vi "AlliGator Conditional Menu Items.vi"(6 "Dataset Series?":bool, 7 "Help?":bool, 8 "Error In":errorcluster, 9 "Menu Item Path":string, 10 "Menu Item Tag":string, 11 "menu reference":refnum<k9>) -> (0 "Error Out":errorcluster, 1 "Quit?":bool, 2 "Message":string, 3 "AlliGator Actions":T1[](array[typedef]))   [LabVIEW 2021, in "AlliGator GUI.lvlib"]
doc: "Handles AlliGator menu items that are only responsive when AlliGator is idle."
uses:
  AlliGator GUI.lvlib
  Phasor/Phasor Calibration Type.ctl
  Action Engine/AlliGator Q Element.ctl
  Action Engine/AlliGator Q Event.ctl
  Image/Image Display Event.ctl
  Image/Image Control Refnum.ctl
  <vilib>/Utility/miscctls.llb/LVPoint32TypeDef.ctl
  Graphs/XY Graph/XY Graph Event.ctl
  Files/AlliGator FLI Dataset Type.ctl
  Files/AlliGator Load Dataset Options.ctl
  Files/AlliGator Select Folder Mode.ctl
  Files/AlliGator Folder Selection.ctl
  Files/AlliGator Export Dataset Options.ctl
  Globals, Variables, Constants/AlliGator Variables List.ctl
  Settings/AlliGator Settings List.ctl
  Fits/Decay Convolution/Decay Model.ctl
  Fits/Residual Type.ctl
  Fits/Non-linear Fitting Method v2.ctl
  Fits/Fit Calculation Method.ctl
  Fits/Non-linear Fitting Algorithm.ctl
  Files/Load-Save File Info.ctl
  AlliGator Windows List.ctl
  AlliGator Open Wndow Event Data.ctl
  GUI/Open VI Options.ctl
  Settings/AlliGator Settings Event.ctl
  Settings/AlliGator Settings Window Messages.ctl
  7dfe82a0-ef7a-4bbc-96a2-555d14fb2b04.vi
  Arrays/Signed Array Index.vi
  Variant/Variant to Data/Variant to Boolean.vi
  Action Engine/AlliGator Action Engine.lvlib
  Files/AlliGator Files.lvlib
  Globals, Variables, Constants/AlliGator Globals, Variables & Constants.lvlib
  Variant/Variant to Data/Variant to Data.lvlib
  Phasor/Phasor.lvlib
  Files/Files.lvlib
  Image/Image.lvlib
  Strings/Strings.lvlib
  Python Plugins API/AlliGator Python Plugins.lvlib
  Sound/Sound.lvlib
  Graphs/XY Graph/XY Graph Add-Ons.lvlib
  Settings/AlliGator Settings.lvlib
  Fits/Fits.lvlib
  GUI/GUI.lvlib
  Scripts/AlliGator Scripts.lvlib
  Fits/IRF(X)PSED/Fit Weights Type v2.ctl
  Fits/IRF(X)PSED/Decay Fit Options v4.ctl
panel:
  in  "Calibration Type":T3
  # "see the AlliGator License on the block diagram (Ctrl+E or Window:Show Block Diagram)"
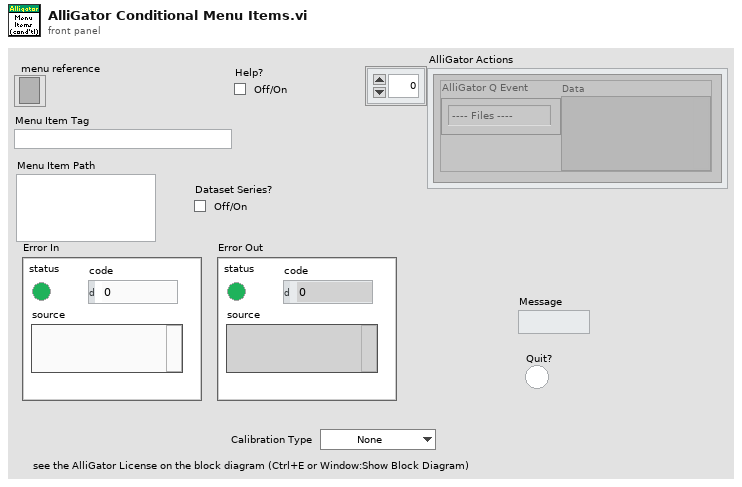
[diagram p1: front panel]
types:
  T1 = typedef "AlliGator Action Engine.lvlib/AlliGator Q Element.ctl" = cluster{"AlliGator Q Event":T2, "Data":variant}
  T2 = typedef "AlliGator Action Engine.lvlib/AlliGator Q Event.ctl" = enum16{"---- Files ----", "Files:Set Batch Export Files To Save", "Files:Set Dataset Loading & Pre-processing Options", "Files:Check #Frames in Dataset", "Files:Increment Frame Index", "Files:Open Mask Image", "Files:Open White Light Image", "Files:Open Single Dataset", "Files:New Folder of Folders Selected", "Files:Load File (all Types)_Scriptable", "Files:Move Flattened Series to Folders Series", "Files:Select Folder", "Files:Load FLI Dataset", "Files:Load Swiss SPAD 1 Dataset", "Files:Load Swiss SPAD 2 Dataset", "Files:Load .sdt FLI Dataset", "Files:Load .ptu FLI Dataset", "Files:Load .bin FLI Dataset", "Files:Load Single Gate Image Folder", "Files:Load I/m/phi Dataset (deprecated)", "Files:Load Single Image", "Files:Subtract Background File", "Files:Export FLI Dataset", "Files:Load HDF5 FLI Dataset", "Files:Set Destination File Path", "Files:Save Mask Image", "Files:Batch Conversion", "Files:New Folder Selected", "Files:Close FLI Dataset", "Files:Close FLI Dataset Series", "Files:Close White Light Image", "Files:Close Mask Image", "---- FLI Dataset ----", "FLI Dataset:Channel Arithmetic", "FLI Dataset:Export Average Lifetime Map as ASCII", "FLI Dataset:Export User-Defined Quantity Map as ASCII", "FLI Dataset:Python Function FLI Dataset Event", "FLI Dataset:ROI Analysis", "FLI Dataset:Tilted Logistic Square Gated IRF Characteristics Map", "FLI Dataset:Logistic Square Gated IRF Characteristics Map", "FLI Dataset:Square Gated IRF Characteristics Map", "FLI Dataset:Multi-ROI Single-Pixel Phasor Analysis", "FLI Dataset:Multi-ROI Single-Pixel NLSF Analysis", "FLI Dataset:All ROIs IRF Extraction", "FLI Dataset:All ROIs Decay Fit Non-Interactive (Fast + Individual IRF)", "FLI Dataset:All ROIs Phasor Analysis", "FLI Dataset:All ROIs Decay Fit", "FLI Dataset:Fluorescence Decay Statistics", "FLI Dataset:Update Decay Statistics Graph", "FLI Dataset:Get Decay from ROI", "FLI Dataset:All ROIs Average Lifetimes", "FLI Dataset:Save/Load Local IRFs", "FLI Dataset:Clear Local IRFs", "FLI Dataset:Phasor Calibration Maps (# Gates Series) Script", "FLI Dataset:Calibrated Phasor Map Series", "---- FLI Dataset Series ----", "FLI Dataset Series:Sum All Datasets in Series", "FLI Dataset Series:Add Dataset to Accumulated Dataset", "FLI Dataset Series:Display Accumulated Dataset", "FLI Dataset Series:Clear Dataset Series Sum", "FLI Dataset Series:Time-Series Analysis (NLSF)", "FLI Dataset Series:Time-Series Analysis (Phasor)", "---- Image ----", "Image:Update Image Profile Plots", "Image:Image Histogram Cursor Move", "Image:Image Histogram", "Image:Image Contrast", "Image:Set Image Histogram Cursor Move Flag", "Image:Clear Image Overlay", "Image:Use ROI as Search Area", "Image:Set ROI Diameter", "Image:Save Image Data as TIFF", "Image:Save Displayed Image with Overlay", "Image:Save Image Overlay Only", "Image:Save Image as Hot Pixel Mask", "Image:Change Source Image Color Palette", "Image:Copy Image to Clipboard", "Image:Source Image ROI Selection", "Image:Delete All ROIs", "Image:Delete All Unselected ROIs", "Image:Delete ROI", "Image:Merge All ROIs", "Image:Store ROI", "Image:Source Image ROI Storage", "Image:Export ROI Description to Notebook", "Image:Save ROI", "Image:Load ROI", "Image:Paste ROI Definition", "Image:Clear ROI", "Image:Identify ROIs in Mask Image", "Image:Create Complementary ROI", "Image:Create Contour ROI", "Image:Create ROI(s) from Pixels with Peak above Min_Scriptable", "Image:Create ROI(s) from Pixels with Intensity above Min_Scriptable", "Image:Compute ROI Statistics", "Image:Delete ROI(s) based on ROI Characteristics", "Image:Create ROI Grid", "Image:ROI to Individual Pixel ROIs", "Image:Python Function Source Image Event", "Image:Show Phasor Calibration Map ROI Centers", "Image:Convert ROI to Mask Image", "Image:Mouse Move", "Image:Mouse Up", "Image:Set Source Image Mouse Move Flag", "Image:Add Scale Bar Overlay", "Image:Delete Existing ROIs Option", "Image:Overlay ROI Median", "Image:Check Current ROI", "Image:Update True Pixel Value", "---- Decay ----", "Decay:Clear IRF/Reference Plot", "Decay:Add Decay to Graph", "Decay:Smoothen Plot", "Decay:Smoothen Plot Tail", "Decay:Average Selected Plots", "Decay:Extract IRF", "Decay:Optimal IRF Extraction", "Decay:Threshold IRF", "Decay:Fit to Model IRF", "Decay:Fit IRF to Square Gate", "Decay:Fit IRF to Logistic Square Gate", "Decay:Fit IRF to Tilted Logistic Square Gate", "Decay:Create Bounding Cursors Set", "Decay:Export Bounding Cursors Definition to Notebook", "Decay:Denoise Plot", "Decay:Compute Cumulative Function", "Decay:Use as Reference Decay", "Decay:Show Reference Decay/IRF", "Decay:Extrapolate Decay", "Decay:Create Head & Tail Bounding Cursors", "Decay:Store Cursor-defined Head & Tail Fractions", "Decay:Rebin Plot", "Decay:1-Normalize Decay", "Decay:[0-1]-Normalize Plot", "Decay:Straighten Decay", "Decay:Shift Decay", "Decay:Fold Decay", "Decay:Fit Decay", "Decay:Global Fit of Selected Decays", "Decay:Post Global Fit Script", "Decay:Add Global Fit Parameters to Graph", "Decay:Add Decay Parameter(s) to Plot (Graph)", "Decay:Export Decay to Phasor Graph", "Decay:Compute Average Lifetime", "Decay:Plot Convolution", "Decay:Graph Tip Strip Update", "---- Decay Statistics ----", "Decay Statistics:Tip Strip Update", "---- Intensity Time Trace ----", "Intensity Time Trace:Use File Timestamp", "Intensity Time Trace:Load Intensity Corrections File", "Intensity Time Trace:Clear Intensity Corrections File", "Intensity Time Trace:Tip Strip Update", "---- Phasor Plot ----", "Phasor Plot:Build Phasor Plot", "Phasor Plot:Change Phasor Plot Color Palette", "Phasor Plot:Adjust Phasor Plot Display Range", "Phasor Plot:Highlight Image ROI in Phasor Plot", "Phasor Plot:Save Phasor Plot Image with Overlay", "Phasor Plot:Export Complex Phasor Map", "Phasor Plot:Export Phasor Ratio Map", "Phasor Plot:Export Average Lifetime Map", "Phasor Plot:Compute Phase Lifetime Histogram", "Phasor Plot:Compute Phasor Ratio Histogram", "Phasor Plot:Compute Phase Lifetime vs Intensity Scatter Plot", "Phasor Plot:Weber 2-Component Decomposition", "Phasor Plot:Update Phasor Color Map Vertices", "Phasor Plot:Clear Phasor Overlay", "Phasor Plot:Use Segment Extremities as References", "Phasor Plot:Use UC/Segment Intersections as References", "Phasor Plot:Use UC/Principal Axis Intersections as References", "Phasor Plot:Use UC/Linear Fit Intersections as References", "Phasor Plot:Update Phasor Plot Reference", "Phasor Plot:Show Local Phasor Info in Phasor Plot", "Phasor Plot:Update Phasor Plot State", "Phasor Plot:Phasor Plot ROI Storage", "Phasor Plot:Phasor Plot ROI Selection", "Phasor Plot:Python Function Phasor Plot Event", "Phasor Plot:Overlay Phasor ROI, Ratio or Map in Source Image", "Phasor Plot:Compute Decay of Selected Phasors", "Phasor Plot:Phasor at Image Pixel", "Phasor Plot:Mouse Move", "Phasor Plot:Mouse Up", "Phasor Plot:Display Range Mouse Move", "Phasor Plot:Set Mouse Move Flag", "Phasor Plot:Update True Phasor Plot Value", "---- Phasor Graph ----", "Phasor Graph:Get Phasor Value", "Phasor Graph:Create New Phasor Plot Dialog", "Phasor Graph:Update Last Phasor Value", "Phasor Graph:Update Phasor (m, phi)", "Phasor Graph:Remove Single Phasor from Plot", "Phasor Graph:Add Single Phasor to Plot", "Phasor Graph:Remove Phasor Plot", "Phasor Graph:Remove Selected Phasor Plots", "Phasor Graph:Clear Phasor Data", "Phasor Graph:Clear Phasor Graph", "Phasor Graph:Cursor Move", "Phasor Graph:Draw Cursor Connecting Line", "Phasor Graph:Clear Cursor Connecting Line", "Phasor Graph:Find UC Intersection", "Phasor Graph:Use UC/Cursor-Defined Line Intersections", "Phasor Graph:Use Selected Plots Fitted Line/UC Intersections", "Phasor Graph:Use Selected Plots Principal Axis/UC Intersections", "Phasor Graph:Show Single Phasor", "Phasor Graph:Save Single Phasor Plot", "Phasor Graph:Save All Phasor Plots", "Phasor Graph:Load Phasor Plot(s)", "Phasor Graph:Phasor Multiplication", "Phasor Graph:Compute Average Phasor", "Phasor Graph:Compute Multiple Average Phasors (Selected Plots)", "Phasor Graph:Export Single Phasor Plot Phase Lifetimes", "Phasor Graph:Parameter 2 vs Parameter 1 Scatter Plot", "Phasor Graph:Use Cursor n Location", "Phasor Graph:Set Reference n to Current Phase Lifetime Value", "Phasor Graph:Set Reference n to Lifetime Value", "Phasor Graph:Set Cursor n Location", "Phasor Graph:Save Phasor Graph Image", "Phasor Graph:Update SEPL Plot", "Phasor Graph:Export Single Phasor Plot Data", "Phasor Graph:Export Selected Phasor Plots Data", "Phasor Graph:Python Function Phasor Graph Event", "Phasor Graph:Tip Strip Update", "---- Calibration ----", "Calibration:Set Calibration Type", "Calibration:Load/Save Phasor Calibration", "Calibration:Load/Save Phasor Calibration Series", "Calibration:Load/Save Phasor Calibration Map", "Calibration:Use as Calibration", "Calibration:Compute Optimal Calibration from Phasor References", "Calibration:Clear Phasor Calibration", "Calibration:Single Phasor Calibration Information", "Calibration:Use as Calibration Series", "Calibration:Use as Calibration Map", "Calibration:Clear Calibration Series", "Calibration:Phasor Calibration Series Information", "Calibration:Clear Calibration Map", "Calibration:Phasor Calibration Map Information", "Calibration:Apply Phasor Calibration", "Calibration:Update Single Plot Calibration", "Calibration:Update Multiple Plots Calibration", "Calibration:Clear Single Plot Calibration", "Calibration:Clear All Plots Calibrations", "Calibration:Clear Plot(s) Calibration(s)?", "---- Phasor Ratio ----", "Phasor Ratio:Clear Reference n", "Phasor Ratio:Toggle Selected Plot(s)  Lock to Reference 1", "Phasor Ratio:Use as Reference n", "Phasor Ratio:Send Reference n to Notebook", "Phasor Ratio:Toggle Selected Plot(s)  Lock to Reference 2", "Phasor Ratio:Compute Phasor Ratio at Mouse Location", "Phasor Ratio:Compute Phasor Plot's Average Phasor Ratio", "Phasor Ratio:Compute Time-Series Phasor Ratios", "Phasor Ratio:Fit Line to Phasor Ratio Plot", "Phasor Ratio:Save References", "Phasor Ratio:Load References", "Phasor Ratio:Update Phasor Reference 1", "Phasor Ratio:Update Phasor Reference 2", "Phasor Ratio:Move Cursor n to Reference n", "Phasor Ratio:Use as Phasor Reference 1 Lifetime", "Phasor Ratio:Use as Phasor Reference 2 Lifetime", "Phasor Ratio:Export Phasor Ratio Map as ASCII", "Phasor Ratio:Tip Strip Update", "---- Lifetime & Other Parameters Graph ----", "Lifetime:Compute Sliced Mean, SDV and CV Plots", "Lifetime:Plot Decay Shifts", "Lifetime:Plot Histogram", "---- Decay Fit Parameter Map ----", "Decay Fit Parameter Map:Export ROI NLSF Data as ASCII", "Decay Fit Parameter Map:Set Decay Fit Parameter Map Selection", "Decay Fit Parameter Map:Build Decay Fit Parameter Map", "Decay Fit Parameter Map:Change Decay Fit Parameter Map Color Palette", "Decay Fit Parameter Map:Export Decay Fit Parameter Map Data as ASCII", "Decay Fit Parameter Map:Export All Decay Fit Parameter Maps Data as ASCII", "Decay Fit Parameter Map:Selected Parameter Scatterplot", "Decay Fit Parameter Map:Parameter 2 vs Parameter 1 Scatterplot", "Decay Fit Parameter Map:Save Decay Fit Parameter Map Image", "Decay Fit Parameter Map:Save-Load IRFs & Fit Data", "Decay Fit Parameter Map:Update Local Decay Plots", "Decay Fit Parameter Map:Python Function Decay Fit Parameters Map Event", "Decay Fit Parameter Map:Overlay Decay Fit Parameter Map in Source Image", "Decay Fit Parameter Map:Selected Parameter vs Intensity Scatterplot", "Decay Fit Parameter Map:Mouse Up", "Decay Fit Parameter Map:Mouse Move", "Decay Fit Parameter Map:Display Range Mouse Move", "Decay Fit Parameter Map:Change Map Resolution", "Decay Fit Parameter Map:Variance Significance Maps", "Decay Fit Parameter Map:Fit Result Constraints Window", "---- Parameter Map ----", "Parameter Map:Export ROI Parameters Data as ASCII", "Parameter Map:Delete Parameter Map Set", "Parameter Map:Update Parameter List", "Parameter Map:Build Parameter Map", "Parameter Map:Change Parameter Map Color Palette", "Parameter Map:Export Parameter Map Data as ASCII", "Parameter Map:Export All Parameter Maps Data as ASCII", "Parameter Map:Selected Parameter Scatterplot", "Parameter Map:Parameter 2 vs Parameter 1 Scatterplot", "Parameter Map:Selected Parameter vs Intensity Scatterplot", "Parameter Map:Save Parameter Map Image", "Parameter Map:Save-Load IRFs & Parameter Maps (TODO)", "Parameter Map:Set Parameter Map Selection", "Parameter Map:Python Function Parameter Map Event", "Parameter Map:Overlay Parameter Map in Source Image", "Parameter Map:Update Local Decay Plots", "Parameter Map:Mouse Up", "Parameter Map:Mouse Move", "Parameter Map:Display Range Mouse Move", "---- Generic Graph ----", "Generic Graph:Generic XY Graph Event", "Generic Graph:Python Function XY Graph Event", "Generic Graph:New Plot", "Generic Graph:Save Plot", "Generic Graph:XY Plot Histogram", "Generic Graph:Set XY Graph Plot Name", "Generic Graph:Set Last Cursor Style", "Generic Graph:Tip Strip Update", "---- GUI ----", "GUI:Start Script", "GUI:Type of Displayed Image Changed", "GUI:Gate Image Slide Changed", "GUI:Show Busy Icon", "GUI:Show Busy Icon & Abort Button", "GUI:Hide Busy Icon", "GUI:Hide Busy Icon & Abort Button", "GUI:Abort", "GUI:End Script", "GUI:Start Timing", "GUI:End Timing", "GUI:Set State Indicator", "GUI:Send Parameters JSON Strings to Clipboard", "GUI:Set Gate Step", "GUI:Idle", "GUI:Initialization", "GUI:Quit", "GUI:Increment Dataset Index", "GUI:Set Dataset Index to -1", "GUI:Time Series Slider Moved", "GUI:Time Series Slider Changed", "GUI:Toggle Playback or Loop", "GUI:Playback Script", "GUI:Set Phasor Frequency", "GUI:Open Window", "GUI:Start Test Script", "GUI:End Test Script", "GUI:Set Verbose Mode", "GUI:Set Verbose Settings Mode", "DEBUG"}
  T3 = typedef "Phasor.lvlib/Phasor Calibration Type.ctl" = enum16{"None", "Single Phasor", "Phasor Series", "Phasor Map"}
  T4 = typedef "Image.lvlib/Image Display Event.ctl" = cluster{"Item Tag":string, "Image Control Refnum":T5, "Coords":T6, "Item Path":string}
  T5 = typedef "Image.lvlib/Image Control Refnum.ctl" = refnum<vi>
  T6 = typedef "LVPoint32TypeDef.ctl" = cluster{"Horizontal":i32, "Vertical":i32}
  T7 = typedef "XY Graph Add-Ons.lvlib/XY Graph Event.ctl" = cluster{"Item Tag":string, "XY Graph Refnum":refnum<vi>, "Coords":T6, "Item Path":string}
  T8 = typedef "AlliGator Files.lvlib/AlliGator Load Dataset Options.ctl" = cluster{"FLI Dataset Type":T9, "No Dialog?":bool, "File Path":path}
  T9 = typedef "AlliGator Files.lvlib/AlliGator FLI Dataset Type.ctl" = enum16{"HDF5 FLI Dataset", "Gate Image Folder", ".sdt FLI Dataset (Becker & Hickl)", ".ptu FLI Dataset (PicoQuant)", "SS1 FLI Dataset", "SS2 FLI Dataset", "I/m/phi Dataset", ".bin FLI Dataset (PicoQuant Binned)", ".bin FLI Dataset (Piccolo Binned)", ".mat FLI Dataset"}
  T10 = typedef "AlliGator Files.lvlib/AlliGator Folder Selection.ctl" = cluster{"Folder Selection Mode":T11, "Folder Path":path}
  T11 = typedef "AlliGator Files.lvlib/AlliGator Select Folder Mode.ctl" = enum16{"Select Gate Folder", "Select Folder of Gate Folders", "Select Folder of SwissSPAD 2 Datasets", "Select Folder of .sdt FLI Datasets (Becker & Hickl)", "Select Folder of .ptu FLI Datasets (PicoQuant)", "Select Folder of .bin FLI Datasets (PicoQuant Binned)", "Select Folder of .bin FLI Datasets (Piccolo Binned)", "Select Folder of HDF5 FLI Datasets"}
  T12 = typedef "AlliGator Files.lvlib/AlliGator Export Dataset Options.ctl" = cluster{"Destination File Type":string, "Dialog?":bool}
  T13 = typedef "AlliGator Globals, Variables & Constants.lvlib/AlliGator Variables List.ctl" = enum16{"---- GUI ----", "GUI:Initialization Status", "GUI:State Indicators Refnum", "GUI:Original AlliGator Menu Items", "GUI:Current Action Loop State", "GUI:Script in progress", "GUI:Playback", "GUI:Loop Playback", "GUI:Search ROI Used", "GUI:Search ROI", "Decay Graph Max Legend Size", "Intensity Graph Max Legend Size", "Decay Statistics Graph Max Legend Size", "Phasor Graph Max Legend Size", "Phasor Ratio Graph Max Legend Size", "Lifetime Graph Max Legend Size", "---- Files ----", "Files:Export Dataset Frames as Individual Files", "Files:Show Batch Export Help Balloons", "Files:Frames in Dataset", "Files:ptu File Frame Start Indices", "Files:Current Frame in Dataset", "Files:Current Frame Timestamp", "Files:Dataset Loaded", "Files:Dataset Metadata", "Files:Dataset Channel", "Files:Dataset Data Description", "Files:Background Dataset Metadata", "Files:Background Dataset Channel", "Files:Background Dataset Data Description", "Files:Background File Subtraction", "Files:Background File Path", "Files:Background File Pile-up Correction", "Files:Background File Pixel Well Capacity", "Files:Background File Scaling Factor", "Files:Current Dataset Load Settings", "Files:Dataset Path", "Files:ICCD-specific Information", "Files:Macrotime Gate Separation", "------ Python Plugins ------", "Python Plugins:Information", "Python Plugins:Python Session", "Python Plugins:Valid Python Session?", "---- Source Image ----", "Source Image:ROIs", "Source Image:Current ROI", "Source Image:ROI Event Refnum", "X_Source Image:Display Range", "X_Source Image:Palette Information", "X_Source Image:Type of Displayed Image", "X_Time Gate Slider", "Source Image:Palette List", "Source Image:Scale", "Source Image:ROI Overlay Color", "Source Image:Overlay to Erase", "Source Image:Is Displayed Image Accumulated", "Source Image:White Light Image Modified", "Source Image:Mask Image Modified", "---- Image Profile Window ----", "Image Profile:Window Event Refnum", "Image Profile:IntensityType", "Image Profile:Intensity Average Type", "Image Profile:Intensity-weighted SDV", "Image Profile:Box Profile Type", "Image Profile:Window Open", "Image Profile:Plotted Fit Parameter", "------ Phasor Graph -------", "Phasor Graph:Show Line", "---- Phasor Plot ---", "Phasor Plot:Parameters Changed", "Phasor Plot:FLI Dataset Modified since last Calculation", "Phasor Harmonics Data", "Selected Phasor Harmonics", "Phasor Harmonic Manager Event Refnum", "Phasor Plot:ROIs", "Phasor Plot:Current ROI", "Phasor Plot:ROI Event Refnum", "Phasor Plot:Image Reference Points", "Phasor Plot:Computed", "Phasor Plot:Palette Information", "Phasor Plot:Palette List", "Phasor Plot:Phasor Ratio Palette Information", "Phasor Plot:Phasor Ratio Palette List", "Phasor Plot:Image Scale", "Phasor Plot:Image Overlay to Erase", "Phasor Plot:Image Elements to Update", "Phasor Plot:Current Calculation Parameters", "Phasor Plot:Current Calibration Options", "Phasor Plot:Reset Cumulated Phasor Plot", "Phasor Plot:Reference 1", "Phasor Plot:Lifetime Reference 1", "Phasor Plot:Reference 1 Frequency", "Phasor Plot:Reference 2", "Phasor Plot:Lifetime Reference 2", "Phasor Plot:Reference 2 Frequency", "---- Decay Analysis ----", "Number of Selected Decays to Fit", "LS Fit Results", "LAR Fit Results", "BS Fit Results", "Last Decay Max - Min", "Best Fit Parameters", "Best Fit Parameter Names", "Actual Size X", "Actual Size Y", "Binning X", "Binning Y", "Actual # Gates", "Dataset Number", "Gates to...", "Gates Skipped", "Gates to keep", "Gate Step", "Gate Separation", "Reversed Gates", "Pile-up Correction", "Pixel Well Capacity", "Background Subtracted", "Background Subtraction Method", "Background Definition Range", "Background File (deprecated)", "Number of Dataset Accumulated", "Array of Accumulated Dataset Paths", "Do Averaged Datasets", "Destination File Path", "Process Plot Target", "Use 1/D as Phasor Frequency", "---- Decay Fit Parameter Map -----", "Decay Fit Parameter Map:Palette Information", "Decay Fit Parameter Map:Palette List", "Decay Fit Parameter Map:X Resolution", "Decay Fit Parameter Map:Y Resolution", "Decay Fit Parameter Map:Use Decay Fit Result Constraints", "Decay Fit Parameter Map:Decay Fit Result Constraints", "Decay Fit Parameter Map:Decay Fit Result Constraints Applied", "---- Parameter Map ----", "Parameter Map:Palette Information", "Parameter Map:Palette List", "------- Local Decay Window ---------", "Local Decay Graph Window:Event Refnum", "Local Decay Graph Window:Use normalized IRF for convolution", "----- Miscellaneous ----", "Misc:Skippable Dialog Windows Status"}
  T14 = typedef "Fits.lvlib/Decay Fit Options v4.ctl" = cluster{"Show Fit Residuals":bool, "Fit Model":T15, "Residual Type":T16, "Max Decay Percentile":dbl, "Min Decay Percentile":dbl, "Show Full Decay":bool, "Weights":T17, "Fitting Method":T18, "Compute Parameter Uncertainties":bool, "Periodic Boundaries":bool, "Model Calculation":T19, "Period":dbl[unit], "Termination Criteria":cluster{"Max Iterations":i32, "Max Function Calls":i32, "Max Time":dbl[unit], "Function Tolerance":dbl, "Parameter Tolerance":dbl, "Gradient Tolerance":dbl, "Min Lambda":dbl, "Max Lambda":dbl, "Initial Tick Count":u32}, "Offset Resolution":dbl[unit], "Use Local IRF":bool, "Fitting Algorithm":T20, "Show Confidence Interval ":bool, "Confidence Level":dbl}
  T15 = typedef "Fits.lvlib/Decay Model.ctl" = enum16{"1-Exponential", "2-Exponentials"}
  T16 = typedef "Fits.lvlib/Residual Type.ctl" = enum16{"Standard", "Normalized", "Reduced"}
  T17 = typedef "Fits.lvlib/Fit Weights Type v2.ctl" = enum16{"Unweighted", "1/Variance (Neyman)", "1/Variance (Pearson)", "Best of All"}
  T18 = typedef "Fits.lvlib/Non-linear Fitting Method v2.ctl" = enum16{"Least Square", "Least Absolute Residual", "Bisquare", "MLE", "-", "Best of All"}
  T19 = typedef "Fits.lvlib/Fit Calculation Method.ctl" = enum16{"Simulation", "Convolution", "Integration"}
  T20 = typedef "Fits.lvlib/Non-linear Fitting Algorithm.ctl" = enum16{"Levenberg-Marquardt", "Trust-Region Dogleg"}
  T21 = typedef "AlliGator Settings.lvlib/AlliGator Settings List.ctl" = enum16{"GUI:Visible Settings Tab", "GUI:Last Run Version", "Source Image:Use Image Histogram for Contrast", "Source Image:Low Count Pixels Rejection Options", "Source Image:High Count Pixels Rejection Options", "Source Image:Use Image Brightness", "Source Image:Blend Overlay with Image Background", "Source Image:Use Fixed ROI Diameter", "Source Image:ROI Diameter", "Source Image:ROI Center Color", "Source Image:Peak Threshold", "Source Image:Intensity Threshold", "Source Image:Image Binning Options", "Source Image:Image Smoothing Options", "Source Image:Image Histogram Active", "Source Image:Invert Binary Mask", "Source Image:Hot Pixel Removal", "Source Image:Overlay Analyzed ROI Center", "Source Image:Auto-Adjust Contrast", "Source Image:Histogram Lower Percentile", "Source Image:Histogram Upper Percentile", "Source Image:Save Source Image", "Source Image:Scale Bar Options", "Source Image:Image Resolution (Pixel Size)", "Source Image:Flatfield Correction", "Source Image:Show Dead Left Columns Correction", "Source Image:Dead Left Columns Correction", "Source Image:Image Pre-Processing Operations Order", "Source Image:Overlay ROI Median", "Source Image:Median Overlay Color", "Data Information:Gate Width", "Data Information:Nanotime Gate Separation", "Data Information:Macrotime Gate Separation", "Data Information:Gate Step", "Data Information:# Gates", "Data Information:Gate Image Exposure", "Data Information:Gate Image Integration", "Data Information:Gates to Skip", "Data Information:Gates to Keep", "Data Information:Define Gates to", "Data Information:Channel Name", "Data Information:Available Channel Names", "Data Information:Channel Arithmetic", "Data Information:Background File Subtraction", "Data Information:Background File", "Data Information:Background Scaling Factor", "Data Information:Background Pile-up Correction", "Data Information:Background Pixel Well Capacity", "Data Information:Laser Period", "Data Information:SYNC Period", "Data Information:Pile-up Correction", "Data Information:Pixel Well Capacity", "Data Information:Dataset Scaling Factor", "Fluorescence Decay_Decay Pre-Processing:Reverse Gates", "Fluorescence Decay_Decay Pre-Processing:Verbose Decay Pre-Processing", "Fluorescence Decay_Decay Pre-Processing:Use Decay Pre-Processing", "Fluorescence Decay_Decay Pre-Processing:Background Subtraction", "Fluorescence Decay_Decay Pre-Processing:Background Definition Range", "Fluorescence Decay_Decay Pre-Processing:Baseline Subtraction Method", "Fluorescence Decay_Decay Pre-Processing:Decay Pre-Processing Operations Order", "Fluorescence Decay_Decay Pre-Processing:Smoothing Parameter", "Fluorescence Decay_Decay Pre-Processing:Shift Decay", "Fluorescence Decay_Decay Pre-Processing:Decay Shift Parameters", "Fluorescence Decay_Decay Pre-Processing:Fold Decay", "Fluorescence Decay_Decay Pre-Processing:# Folds", "Fluorescence Decay_Decay Pre-Processing:1-Normalize Decay", "Fluorescence Decay_Decay Pre-Processing:[0-1]-Normalize Decay", "Fluorescence Decay_Decay Pre-Processing:Smoothen Decay", "Fluorescence Decay_Decay Pre-Processing:Extrapolate Decay", "Fluorescence Decay_Decay Pre-Processing:Use Periodicity", "Fluorescence Decay_Decay Pre-Processing:Use Cursors", "Fluorescence Decay_Decay Pre-Processing:Tail Fraction", "Fluorescence Decay_Decay Pre-Processing:Head Fraction", "Fluorescence Decay_Decay Pre-Processing:Additional Points", "Fluorescence Decay_Decay Pre-Processing:Straighten Decay", "Fluorescence Decay_Decay Pre-Processing:Constant Background", "Fluorescence Decay_Decay Pre-Processing:Pixel-Normalize Decay", "Fluorescence Decay_Advanced Analysis:Extract IRF instead of Decay", "Fluorescence Decay_Advanced Analysis:IRF Extraction Options", "Fluorescence Decay_Advanced Analysis:IRF Optimization Options", "Fluorescence Decay_Advanced Analysis:Square Pulse Options", "Fluorescence Decay_Advanced Analysis:IRF Order", "Fluorescence Decay_Advanced Analysis:IRF Time Constants", "Fluorescence Decay_Advanced Analysis:Wavelet Analysis Options", "Fluorescence Decay_Advanced Analysis:Average Lifetime Options", "Fluorescence Decay_Fit Options:Fit Options", "Fluorescence Decay_Fit Options:Use Legacy Fitting Approach", "Fluorescence Decay_Fit Options:Use Data Information Laser Period", "Fluorescence Decay_Fit Parameters:Displayed Fit Parameters", "Fluorescence Decay_Fit Parameters:Fit Parameter Constraints", "Fluorescence Decay_Fit Parameters:Export Tabulated Results", "Fluorescence Decay_Fit Parameters:MLE Baseline Offset Type", "Fluorescence Decay_Fit Parameters:MLE Baseline Offset", "Fluorescence Decay_Fit Parameters:Guess Parameter Names", "Fluorescence Decay_Fit Parameters:Guess Parameter Values", "Fluorescence Decay_Fit Parameters:Guess Parameters Options", "Fluorescence Decay_Fit Parameters:Optimal Offset Selection Criterion", "Fluorescence Decay_Styles:Show Last Decay Only", "Fluorescence Decay_Styles:Decay Graph Color Array", "Fluorescence Decay:Decay Graph Active", "Fluorescence Decay Statistics:Min Peak Value", "Fluorescence Decay Statistics:Reject Low Decay Peak Pixels", "Fluorescence Decay Statistics:Reject High Decay Peak Pixels", "Fluorescence Decay Statistics:Max Peak Value", "Time Traces:Use File Timestamp", "Time Traces:Time Step", "Time Traces:Use Intensity Correction File", "Time Traces:Intensity Correction File", "Phasor Plot:Phasor Plot Smoothing Options", "Phasor Plot:Phasor Plot Size", "Phasor Plot:Phasor Plot Graphics Options", "Phasor Plot:Cumulative Phasor Plot", "Phasor Plot:Use Phasor Brightness", "Phasor Plot:Blend Overlay with Phasor Background", "Phasor Plot:Save Phasor Plot", "Phasor Plot:Show References", "Phasor Plot:Phasor Ratio Decay Range", "Phasor Plot:Exponential Fading", "Phasor Plot:Phasor Ratio Reference Colors", "Phasor Plot:Reference Radius", "Phasor Plot:Show Color Map Vertices", "Phasor Plot:Phasor Plot Active", "Phasor Plot:Phasor Ratio Color Map Type", "Phasor Plot:Phasor Ratio Color Map", "Phasor Plot:Phasor Ratio Display Range", "Phasor Plot:Selected Image ROI(s)", "Phasor Plot:All Image ROIs", "Phasor Plot:Selected Phasor Plot ROI(s)", "Phasor Plot:All Phasor Plot ROIs", "Phasor Plot:Phasor Ratio Color-Coded Quantity", "Phasor Plot:Store Phasor Harmonics", "Phasor Plot:Draw Reference Segment", "Phasor Plot:User-Defined Quantity", "Phasor Plot:Color Scale High Color", "Phasor Plot:Color Scale Low Color", "Phasor Plot:Intensity-weighted Phasor Plot", "Phasor Graph:Phasor Frequency", "Phasor Graph:Phasor Ratio Type", "Phasor Graph:Pixel-level Phasor Computation", "Phasor Graph:Save Phasor Graph", "Phasor Graph:Phasor Graph Active", "Phasor Graph:Phasor SDV Options", "Phasor Graph:Intensity-weighted Phasor Graph", "Phasor Graph:Define Shortest Lifetime as", "Phasor Calibration:Use Backup Calibration if needed", "Phasor Calibration:Backup Calibration Type", "Phasor Calibration:Calibration Type", "Phasor Calibration:Calibration Lifetime", "Phasor Calibration:Calibration Map Algorithm", "Single-Exponential Phasor Locus (SEPL):Gate Parameters", "Single-Exponential Phasor Locus (SEPL):User-defined Gate", "Single-Exponential Phasor Locus (SEPL):User-defined IRF", "Single-Exponential Phasor Locus (SEPL):Phasor Parameters", "Single-Exponential Phasor Locus (SEPL):Decay & IRF Parameters", "Single-Exponential Phasor Locus (SEPL):Display Parameters", "Lifetime Analysis:Decay Analysis Parameters", "Lifetime Analysis:Lifetime Map Active", "Plugins:Python Settings", "Miscellaneous:Verbose Mode", "Miscellaneous:Beep after Script", "Miscellaneous:Saved Image File Format", "Miscellaneous:Exported Gate Image Settings", "Miscellaneous:Include Loading in Timing", "Miscellaneous:Verbose Settings Mode", "Miscellaneous:Histogram Options", "Miscellaneous:Beep on Error", "Miscellaneous:# Logical Processors Used", "Miscellaneous:ROI Description Max Characters", "Miscellaneous:Verbose Error Mode", "Miscellaneous:Transparent Mask Color"}
  T22 = typedef "Files.lvlib/Load-Save File Info.ctl" = cluster{"Load/Save":bool, "File Path":path}
  T23 = typedef "AlliGator GUI.lvlib/AlliGator Open Wndow Event Data.ctl" = cluster{"AlliGator Windows":T24, "Open Window Options":T25}
  T24 = typedef "AlliGator GUI.lvlib/AlliGator Windows List.ctl" = enum16{"AlliGator Window", "Settings Window", "Notebook Window", "Dataset Information Window", "Source Image ROI Manager Window", "Phasor Plot ROI Manager Window", "Phasor Harmonic Manager Window", "Histogram Window", "Image Profile Window", "Local Decay Window", "About Window", "Batch Conversion Window", "Shot Noise Influence on Average Lifetime", "Fit Method Benchmark", "Camera Noise Influence on Lifetime", "AlliGator Alias Definition", "Fit Result Constraints Window"}
  T25 = typedef "GUI.lvlib/Open VI Options.ctl" = cluster{"Bring To Front (T)":bool, "Start Hidden? (F)":bool, "Activate? (T)":bool}
  T26 = typedef "AlliGator GUI.lvlib/AlliGator Ctrl Refnums.ctl" = cluster{"Other AlliGator Ctrl Refnums":T27, "Phasor Plot Ctrl Refnums":T28, "Phasor Graph Ctrl Refnums":T29, "Dataset Control Refnums":T30, "Registered Events Ctrl Refnums":T31, "Image Histogram Ctrl Refnums":T32, "Decay Fit Map Ctrl Refnums":T33, "Parameter Map Ctrl Refnums":T34}
  T27 = typedef "AlliGator GUI.lvlib/AlliGator Other Ctrl Refnums.ctl" = cluster{"State Indicators":refnum<vi>, " Progress Bar":refnum<vi>, "Decay Graph Active":refnum<vi>, "Decay Statistics Bin":refnum<vi>, "Time Step":refnum<vi>, "Use File Timestamp":refnum<vi>, "Tab Control":refnum<vi>, "CPU":refnum<vi>, "Abort Fit":refnum<vi>, "Dataset File/Folder Path":refnum<vi>, "Abort ROI Creation":refnum<vi>, "Event LED":refnum<vi>, "Dataset File/Folder Path 2":refnum<vi>, "Dataset File/Folder Path 3":refnum<vi>, "Dataset File/Folder Path 4":refnum<vi>, "Dataset File/Folder Path 5":refnum<vi>, "Dataset File/Folder Path 6":refnum<vi>, "Dataset File/Folder Path 7":refnum<vi>, "Dataset File/Folder Path 8":refnum<vi>, "Dataset File/Folder Path 9":refnum<vi>, "Dataset File/Folder Path 10":refnum<vi>, "Dataset File/Folder Path 11":refnum<vi>}
  T28 = typedef "AlliGator GUI.lvlib/AlliGator Phasor Plot Ctrl Refnums.ctl" = cluster{"Phasor Ratio":refnum<vi>, "Modulus Lifetime":refnum<vi>, "Phasor at cursor (m, phi)":refnum<vi>, "Phase Lifetime":refnum<vi>, "Phasor at cursor (g, s)":refnum<vi>, "Phasor Plor Average Lifetime":refnum<vi>, "Phasor Plot Active":refnum<vi>, "Save Phasor Plot":refnum<vi>, "Image Overlay Color":refnum<vi>, "Phasor Plot Color Scale":refnum<vi>, "Reference 1 Button":refnum<vi>, "Reference 2 Button":refnum<vi>, "True Phasor Plot Value":refnum<vi>}
  T29 = typedef "AlliGator GUI.lvlib/AlliGator Phasor Graph Ctrl Refnums.ctl" = cluster{"Phasor Ratio":refnum<vi>, "Modulus Lifetime":refnum<vi>, "Phasor at cursor (m, phi)":refnum<vi>, "Phase Lifetime":refnum<vi>, "Phasor at cursor (g, s)":refnum<vi>, "Phasor Graph Average Lifetime":refnum<vi>, "Phasor Graph Active":refnum<vi>, "Save Phasor Graph":refnum<vi>, "Phasor Frame Slide":refnum<vi>, "Single Step Phasor":refnum<vi>, "Calibration Type":refnum<vi>, "Show Line":refnum<vi>, "Phase Lifetime 1":refnum<vi>, "Phase Lifetime 2":refnum<vi>, "Phasor Graph Frequency":refnum<vi>, "Phasor Reference 1 Control":refnum<vi>, "Phasor Reference 2 Control":refnum<vi>, "Calibration Lifetime":refnum<vi>, "Phase Lifetime SDV":refnum<vi>, "Average Lifetime SDV":refnum<vi>, "Phasor Ratio SDV":refnum<vi>, "Modulus Lifetime SDV":refnum<vi>}
  T30 = typedef "AlliGator GUI.lvlib/AlliGator Dataset Ctrl Refnums.ctl" = cluster{"Current Data":refnum<vi>, "Gate Image Slide":refnum<vi>, "Time Point Slide":refnum<vi>, "Current Time Stamp":refnum<vi>, "Save Image":refnum<vi>, "Displayed Image":refnum<vi>, "Overlay Mode":refnum<vi>, "Phasor Overlay Color":refnum<vi>, "Image Color Scale":refnum<vi>, "Use ROI as Search Area":refnum<vi>, "Source Image ROI Color":refnum<vi>, "True Pixel Value":refnum<vi>}
  T31 = typedef "AlliGator GUI.lvlib/AlliGator Registered Events Ctrl Refnums.ctl" = cluster{"Time Point Slider":refnum<vi>, "Phasor Plot Display Range":refnum<vi>, "Decay Graph":refnum<vi>, "Decay Statistics Graph":refnum<vi>, "Intensity Time Trace":refnum<vi>, "Phasor Graph":refnum<vi>, "Phasor Ratio Graph":refnum<vi>, "Lifetime Graph":refnum<vi>, "Phasor Plot Display":refnum<vi>, "Source Image Display":refnum<vi>, "Decay Fit Parameter Map Display Range":refnum<vi>, "Decay Fit Parameter Map Display":refnum<vi>, "Parameter Map Display Range":refnum<vi>, "Parameter Map Display":refnum<vi>, "Phasor Plot Display Range":refnum<vi>}
  T32 = typedef "AlliGator GUI.lvlib/AlliGator Image Histogram Control Refnums.ctl" = cluster{"Image Histogram":refnum<vi>, "Image Histogram Options":refnum<vi>, "Image Histogram Active":refnum<vi>, "Image Histogram Upper Percentile":refnum<vi>, "Image Histogram Lower Percentile":refnum<vi>, "Auto-Adjust Contrast":refnum<vi>}
  T33 = typedef "AlliGator Decay Fit Parameter Map.lvlib/AlliGator Decay Fit Map Control Refnums.ctl" = cluster{"Decay Fit Parameter Map Color Scale":refnum<vi>, "Decay Fit Parameter":refnum<vi>, "Max Parameter":refnum<vi>, "Min Parameter":refnum<vi>, "Decay Fit Parameter Map Display":refnum<vi>, "Decay Fit Parameter Map Display Range":refnum<vi>, "Decay Parameter Map X":refnum<vi>, "Decay Parameter Map Y":refnum<vi>, "Decay Parameter Map Value":refnum<vi>}
  T34 = typedef "AlliGator Parameter Map.lvlib/AlliGator Parameter Map Control Refnums.ctl" = cluster{"Parameter Map Color Scale":refnum<vi>, "Map Parameter":refnum<vi>, "Max Parameter":refnum<vi>, "Min Parameter":refnum<vi>, "Parameter Map Display":refnum<vi>, "Parameter Map Display Range":refnum<vi>, "Parameter Map Set":refnum<vi>, "Parameter Map X":refnum<vi>, "Parameter Map Y":refnum<vi>, "Parameter Map Value":refnum<vi>}
  T35 = typedef "AlliGator Scripts.lvlib/AlliGator Series Analysis Type.ctl" = enum16{"Current ROI (Fixed)", "All ROIs (Fixed)", "Sequential ROIs"}
  T36 = typedef "AlliGator Settings.lvlib/AlliGator Settings Event.ctl" = cluster{"AlliGator Settings Message":T37, "Sender":string, "Control Label":string, "Data":variant}
  T37 = typedef "AlliGator Settings.lvlib/AlliGator Settings Window Messages.ctl" = enum16{"Idle", "Subscribe", "Unsubscribe", "Refresh Parameter", "Refresh All Parameters", "Quit"}
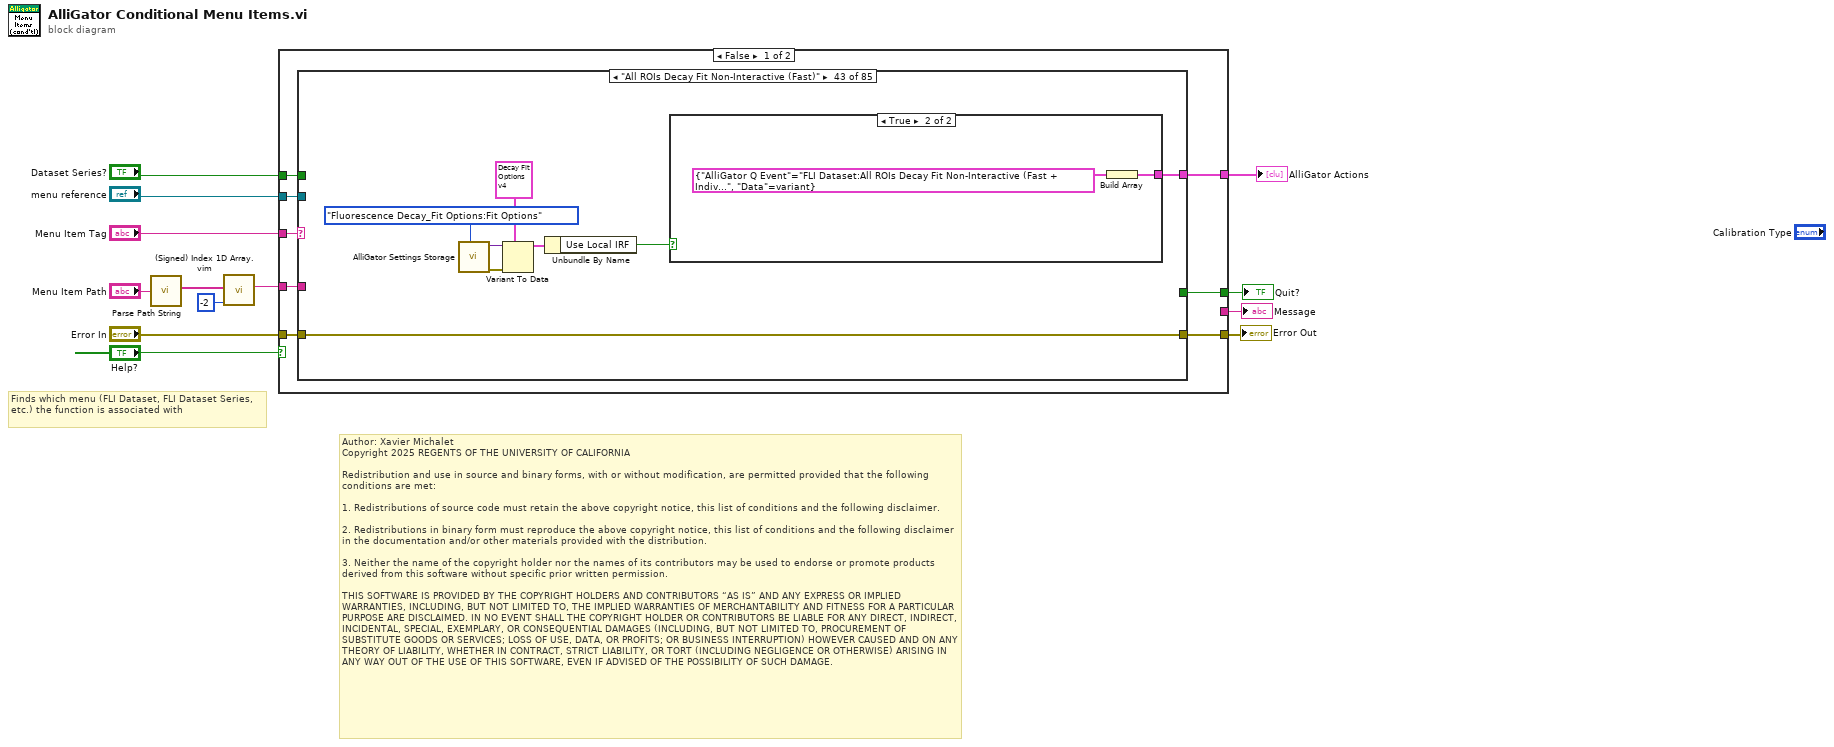
[diagram p0: block diagram]
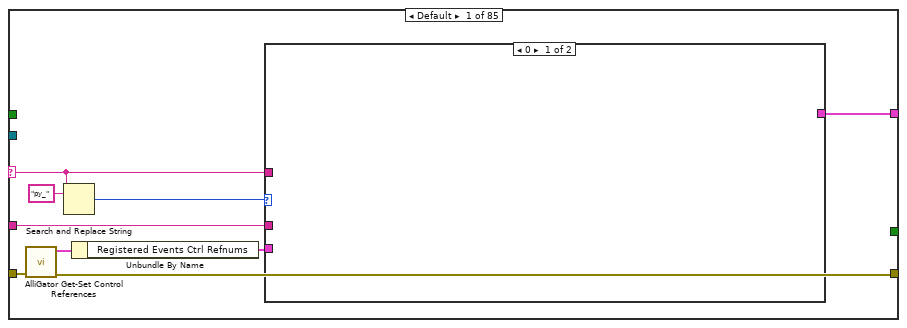
[diagram p2: hidden frame]
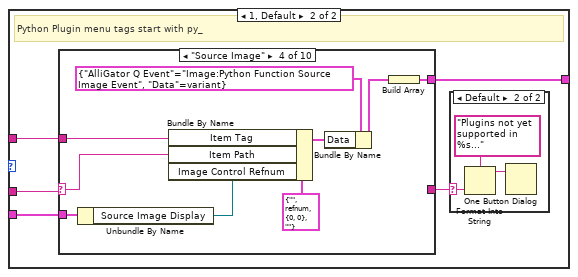
[diagram p3: hidden frame]
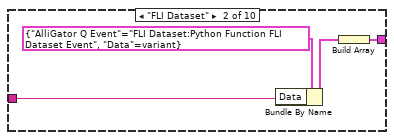
[diagram p6: hidden frame]
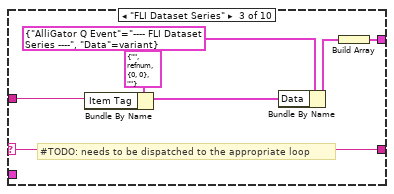
[diagram p7: hidden frame]
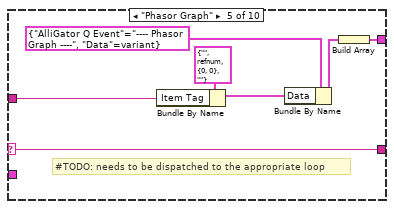
[diagram p8: hidden frame]
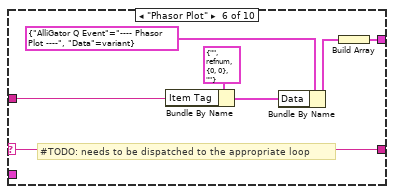
[diagram p9: hidden frame]
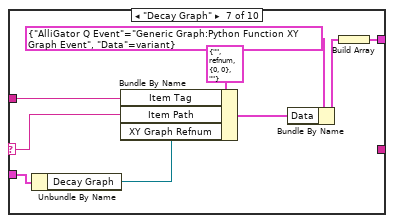
[diagram p10: hidden frame]
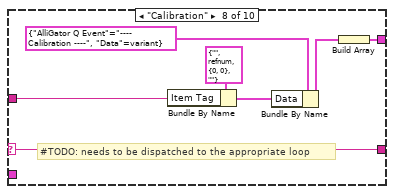
[diagram p11: hidden frame]
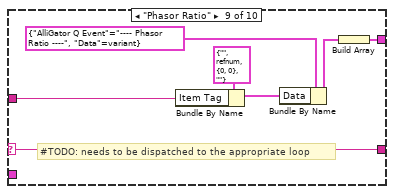
[diagram p12: hidden frame]
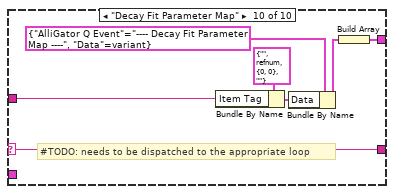
[diagram p13: hidden frame]
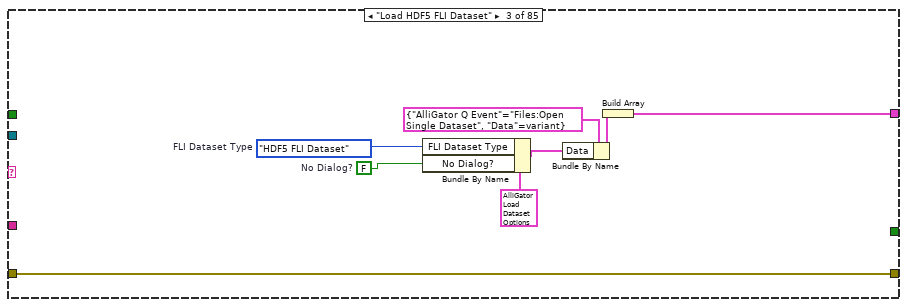
[diagram p15: hidden frame]
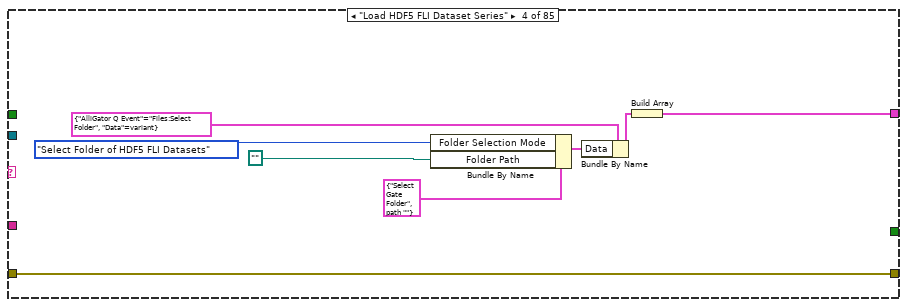
[diagram p16: hidden frame]
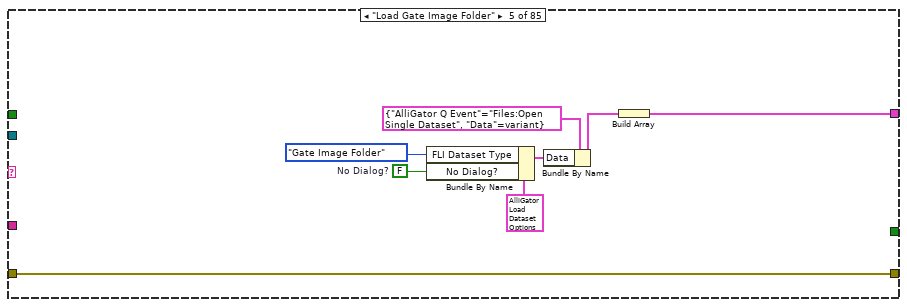
[diagram p17: hidden frame]
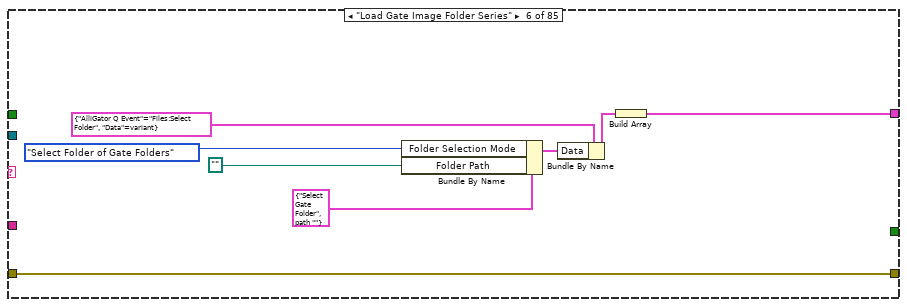
[diagram p18: hidden frame]
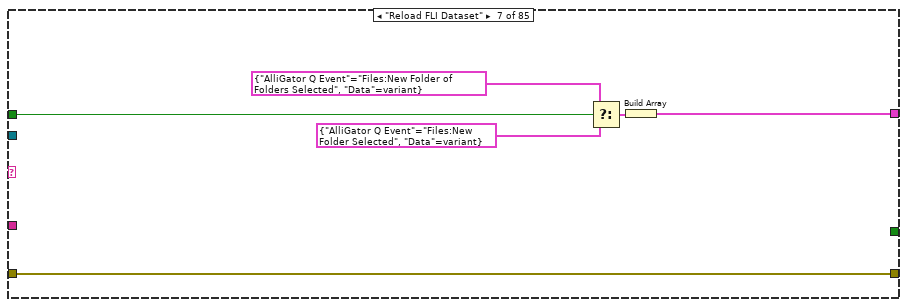
[diagram p19: hidden frame]
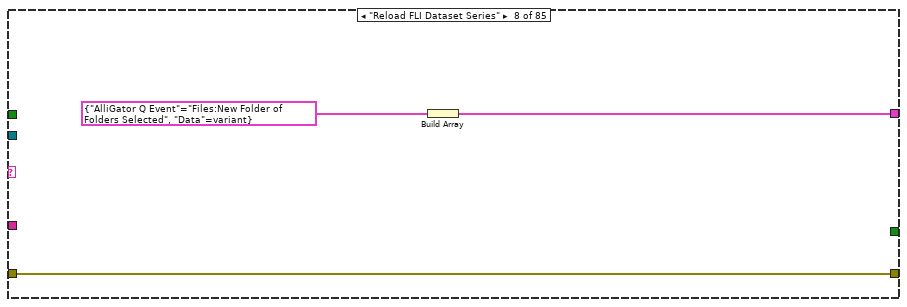
[diagram p20: hidden frame]
diagram:
  # "Author: Xavier Michalet\nCopyright 2025 REGENTS OF THE UNIVERSITY OF CALIFORNIA\n\nRedistribution and use in source and binary forms, with or without modification, are permitted provided that the following conditions are met:\n\n1. Redistributions of source code must retain the above copyright notice, this list of conditions and the following disclaimer.\n\n2. Redistributions in binary form must reproduce the above copyright notice, this list of conditions and the following disclaimer in the documentation and/or other materials provided with the distribution.\n\n3. Neither the name of the copyright holder nor the names of its contributors may be used to endorse or promote products derived from this software without specific prior written permission.\n\nTHIS SOFTWARE IS PROVIDED BY THE COPYRIGHT HOLDERS AND CONTRIBUTORS “AS IS” AND ANY EXPRESS OR IMPLIED WARRANTIES, INCLUDING, BUT NOT LIMITED TO, THE IMPLIED WARRANTIES OF MERCHANTABILITY AND FITNESS FOR A PARTICULAR PURPOSE ARE DISCLAIMED. IN NO EVENT SHALL THE COPYRIGHT HOLDER OR CONTRIBUTORS BE LIABLE FOR ANY DIRECT, INDIRECT, INCIDENTAL, SPECIAL, EXEMPLARY, OR CONSEQUENTIAL DAMAGES (INCLUDING, BUT NOT LIMITED TO, PROCUREMENT OF SUBSTITUTE GOODS OR SERVICES; LOSS OF USE, DATA, OR PROFITS; OR BUSINESS INTERRUPTION) HOWEVER CAUSED AND ON ANY THEORY OF LIABILITY, WHETHER IN CONTRACT, STRICT LIABILITY, OR TORT (INCLUDING NEGLIGENCE OR OTHERWISE) ARISING IN ANY WAY OUT OF THE USE OF THIS SOFTWARE, EVEN IF ADVISED OF THE POSSIBILITY OF SUCH DAMAGE."
  # "Finds which menu (FLI Dataset, FLI Dataset Series, etc.) the function is associated with"
  n1 = call "Parse Path String.vi"("Path in"="Menu Item Path") -> ("Folder Hierarchy"=w6:string[])  [unwired: 4 in, 1 out]
  n2 = call "(Signed) Index 1D Array.vim"("Signed Index"=-2, "Array"=w6) -> ("Array Element"=w4:string)  [unwired: 9 in]
  n3 = case shown="False" "Help?" {
    tunnel: "Menu Item Tag" -> [w21 w523]
    tunnel: [w20 _] -> w12
    tunnel: "menu reference" -> [w19 _]
    tunnel: "Error In" -> [w18 w525]
    tunnel: [w15 w524] -> w9
    tunnel: w4 -> [w17 w522]
    tunnel: [w16 _] -> w3
    tunnel: [_ w521] -> w2
    tunnel: "Dataset Series?" -> [w14 _]
    frame False {
      n4 = case shown="\"All ROIs Decay Fit Non-Interactive (Fast)\"" w21 {
        selector: w21 -> [w26 _ _ _ _ _ _ _ _ _ _ _ _ _ _ _ _ _ _ _ _ _ _ _ _ _ _ _ _ _ _ _ _ _ _ _ _ _ _ _ _ _ _ _ _ _ _ _ w347 _ _ w357 w361 _ _ _ _ _ _ _ _ _ _ _ _ _ _ _ _ w434 _ _ _ _ w464 _ _ _ _ w495 _ _ _ _ _]
        tunnel: [_ _ _ _ _ _ _ _ _ _ _ _ _ _ _ _ _ _ _ _ _ _ _ _ _ _ _ _ _ _ _ _ _ w274 _ _ _ _ _ _ _ _ _ _ _ _ _ _ _ _ _ _ _ _ _ _ _ _ _ _ _ _ _ _ _ _ _ _ _ _ _ _ _ _ _ _ _ _ _ _ _ _ _ _ _] -> w20
        tunnel: w19 -> [_ _ _ _ _ _ _ _ _ _ _ _ _ _ _ _ _ _ _ _ _ _ _ _ _ _ _ _ _ _ _ _ _ _ _ _ _ _ _ _ _ _ _ _ _ _ _ _ _ _ _ _ _ _ _ _ _ _ _ _ _ _ _ _ _ _ _ _ _ w432 _ _ _ _ w466 _ _ _ _ w497 _ _ _ _ _]
        tunnel: [w28 _ w109 w113 w125 w129 w141 w143 w150 w158 w162 w171 w178 w190 w194 w206 w214 w218 w226 T1[] [{"AlliGator Q Event"=enum."Files:Move Flattened Series to Folders Series", "Data"=variant}] ("element") T1[] [{"AlliGator Q Event"=enum."Files:Open White Light Image", "Data"=variant}] ("element") T1[] [{"AlliGator Q Event"=enum."Files:Open Mask Image", "Data"=variant}] ("element") w240 w252 w256 T1[] [{"AlliGator Q Event"=enum."Intensity Time Trace:Load Intensity Corrections File", "Data"=variant}] ("element") T1[] [{"AlliGator Q Event"=enum."Files:Save Mask Image", "Data"=variant}] ("element") T1[] [{"AlliGator Q Event"=enum."Files:Close FLI Dataset", "Data"=variant}] ("element") T1[] [{"AlliGator Q Event"=enum."Files:Close FLI Dataset Series", "Data"=variant}] ("element") T1[] [{"AlliGator Q Event"=enum."Files:Close White Light Image", "Data"=variant}] ("element") T1[] [{"AlliGator Q Event"=enum."Files:Close Mask Image", "Data"=variant}] ("element") T1[] [{"AlliGator Q Event"=enum."Intensity Time Trace:Clear Intensity Corrections File", "Data"=variant}] ("element") T1[] [{"AlliGator Q Event"=enum."DEBUG", "Data"=variant}] ("element") w275 _ _ T1[] [{"AlliGator Q Event"=enum."FLI Dataset:ROI Analysis", "Data"=variant}] ("element") w291 w296 w301 w306 w311 w322 w331 T1[] [{"AlliGator Q Event"=enum."FLI Dataset:Multi-ROI Single-Pixel Phasor Analysis", "Data"=variant}] ("element") T1[] [{"AlliGator Q Event"=enum."FLI Dataset:Multi-ROI Single-Pixel NLSF Analysis", "Data"=variant}] ("element") T1[] [{"AlliGator Q Event"=enum."Decay:Global Fit of Selected Decays", "Data"=variant}] ("element") T1[] [{"AlliGator Q Event"=enum."FLI Dataset:Fluorescence Decay Statistics", "Data"=variant}] ("element") w348 T1[] [{"AlliGator Q Event"=enum."FLI Dataset:Clear Local IRFs", "Data"=variant}] ("element") _ w355 w362 T1[] [{"AlliGator Q Event"=enum."FLI Dataset Series:Sum All Datasets in Series", "Data"=variant}] ("element") w369 w374 T1[] [{"AlliGator Q Event"=enum."FLI Dataset Series:Clear Dataset Series Sum", "Data"=variant}] ("element") _ _ w383 w393 w403 _ T1[] [{"AlliGator Q Event"=enum."FLI Dataset:Phasor Calibration Maps (# Gates Series) Script", "Data"=variant}] ("element") T1[] [{"AlliGator Q Event"=enum."FLI Dataset:Calibrated Phasor Map Series", "Data"=variant}] ("element") T1[] [{"AlliGator Q Event"=enum."FLI Dataset:Square Gated IRF Characteristics Map", "Data"=variant}] ("element") T1[] [{"AlliGator Q Event"=enum."FLI Dataset:Logistic Square Gated IRF Characteristics Map", "Data"=variant}] ("element") T1[] [{"AlliGator Q Event"=enum."FLI Dataset:Tilted Logistic Square Gated IRF Characteristics Map", "Data"=variant}] ("element") _ _ T1[] [{"AlliGator Q Event"=enum."Calibration:Single Phasor Calibration Information", "Data"=variant}] ("element") w439 w446 w453 _ T1[] [{"AlliGator Q Event"=enum."Calibration:Phasor Calibration Series Information", "Data"=variant}] ("element") w470 w477 w484 _ T1[] [{"AlliGator Q Event"=enum."Calibration:Phasor Calibration Map Information", "Data"=variant}] ("element") T1[] [{"AlliGator Q Event"=enum."Image:Show Phasor Calibration Map ROI Centers", "Data"=variant}] ("element") w503 w510 w517] -> w16
        tunnel: w18 -> [w25 w103 w104 w112 w120 w128 w140 w142 w145 w153 w161 w169 w177 w185 w193 w201 w209 w217 w225 w234 w235 w237 w239 w247 w255 w258 w260 w262 w264 w266 w268 w270 w272 w277 w286 w287 w288 w290 w295 w300 w305 w310 w321 w330 w332 w334 w336 w338 w345 w352 w353 w358 w365 w366 w368 w373 w378 w380 w381 w391 w401 w411 w412 w413 w415 w417 w419 w421 w423 w428 w437 w438 w445 w452 w463 w468 w469 w476 w483 w493 w499 w501 w502 w509 w516]
        tunnel: [w24 w103 w104 w112 w120 w128 w140 w142 w145 w153 w161 w169 w177 w185 w193 w201 w209 w217 w225 w234 w235 w237 w239 w247 w255 w258 w260 w262 w264 w266 w268 w270 w272 w276 w286 w287 w288 w290 w295 w300 w305 w310 w321 w330 w332 w334 w336 w338 w344 w352 w353 w358 w365 w366 w368 w373 w378 w380 w381 w391 w401 w411 w412 w413 w415 w417 w419 w421 w423 w428 w437 w438 w445 w452 w463 w468 w469 w476 w483 w493 w499 w501 w502 w509 w516] -> w15
        tunnel: w17 -> [w27 _ _ _ _ _ _ _ _ _ _ _ _ _ _ _ _ _ _ _ _ _ _ _ _ _ _ _ _ _ _ _ _ _ _ _ _ _ _ _ _ _ _ _ _ _ _ _ _ _ _ _ _ _ _ _ _ _ _ _ _ _ _ _ _ _ _ _ _ _ _ _ _ _ _ _ _ _ _ _ _ _ _ _ _]
        tunnel: w14 -> [_ _ _ _ _ _ w138 _ _ _ _ _ _ _ _ _ _ _ _ _ _ _ _ _ _ _ _ _ _ _ _ _ _ _ _ _ _ _ _ _ _ _ _ _ _ _ _ _ _ _ _ _ _ _ _ _ _ _ _ _ _ _ _ _ _ _ _ _ _ _ _ _ _ _ _ _ _ _ _ _ _ _ _ _ _]
        frame Default {
          n5 = call "AlliGator Get-Set Control References.vi"("Error In"=w25) -> ("Error Out"=w24:errorcluster, "AlliGator Ctrl Refnums out"=w23:T26)  [unwired: 9 in]
          n6 = Search and Replace String(input string=w26, search string="py_") -> (number of replacements=w29:i32)  [unwired: 6 in, 3 out]
          n7 = Unbundle By Name(w23) -> ("Registered Events Ctrl Refnums"=w22:T31)
          n8 = case shown="0" w29 {
            tunnel: [_ w35] -> w28
            tunnel: w27 -> [_ w33]
            tunnel: w26 -> [_ w34]
            tunnel: w22 -> [_ w31]
            frame 0 {
            }
            frame 1, Default {
              # "Python Plugin menu tags start with py_"
              n9 = case shown="\"Source Image\"" w33 {
                selector: w33 -> [_ _ w43 w52 w59 w66 w75 w82 w89 w96]
                tunnel: [_ w42 w49 w58 w65 w72 w81 w88 w95 w102] -> w35
                tunnel: w34 -> [_ w39 w44 w53 w60 w67 w77 w83 w90 w97]
                tunnel: [_ _ w43 _ w59 w66 _ w82 w89 w96] -> w32
                tunnel: w31 -> [_ _ _ w51 _ _ w74 _ _ _]
                frame "", Default {
                }
                frame "FLI Dataset" {
                  n10 = Bundle By Name(cluster=T1 {"AlliGator Q Event"=enum."FLI Dataset:Python Function FLI Dataset Event", "Data"=variant}, "Data"=w39) -> (w40:T1)
                  n11 = Build Array(w40) -> (w42:T1[])
                }
                frame "FLI Dataset Series" {
                  # "#TODO: needs to be dispatched to the appropriate loop"
                  n12 = Bundle By Name(cluster=T4 {"Item Tag"="", "Image Control Refnum"=refnum, "Coords"={"Horizontal"=0, "Vertical"=0}, "Item Path"=""} ("Image Event"), "Item Tag"=w44) -> (w46:T4)
                  n13 = Bundle By Name(cluster=T1 {"AlliGator Q Event"=enum."---- FLI Dataset Series ----", "Data"=variant}, "Data"=w46) -> (w47:T1)
                  n14 = Build Array(w47) -> (w49:T1[])
                }
                frame "Source Image" {
                  n15 = Unbundle By Name(w51) -> ("Source Image Display"=w50:refnum<vi>)
                  n16 = Bundle By Name(cluster=T4 {"Item Tag"="", "Image Control Refnum"=refnum, "Coords"={"Horizontal"=0, "Vertical"=0}, "Item Path"=""} ("Image Event"), "Item Tag"=w53, "Item Path"=w52, "Image Control Refnum"=w50) -> (w55:T4)
                  n17 = Bundle By Name(cluster=T1 {"AlliGator Q Event"=enum."Image:Python Function Source Image Event", "Data"=variant}, "Data"=w55) -> (w56:T1)
                  n18 = Build Array(w56) -> (w58:T1[])
                }
                frame "Phasor Graph" {
                  # "#TODO: needs to be dispatched to the appropriate loop"
                  n19 = Bundle By Name(cluster=T4 {"Item Tag"="", "Image Control Refnum"=refnum, "Coords"={"Horizontal"=0, "Vertical"=0}, "Item Path"=""} ("Image Event"), "Item Tag"=w60) -> (w62:T4)
                  n20 = Bundle By Name(cluster=T1 {"AlliGator Q Event"=enum."---- Phasor Graph ----", "Data"=variant}, "Data"=w62) -> (w63:T1)
                  n21 = Build Array(w63) -> (w65:T1[])
                }
                frame "Phasor Plot" {
                  # "#TODO: needs to be dispatched to the appropriate loop"
                  n22 = Bundle By Name(cluster=T4 {"Item Tag"="", "Image Control Refnum"=refnum, "Coords"={"Horizontal"=0, "Vertical"=0}, "Item Path"=""} ("Image Event"), "Item Tag"=w67) -> (w69:T4)
                  n23 = Bundle By Name(cluster=T1 {"AlliGator Q Event"=enum."---- Phasor Plot ----", "Data"=variant}, "Data"=w69) -> (w70:T1)
                  n24 = Build Array(w70) -> (w72:T1[])
                }
                frame "Decay Graph" {
                  n25 = Unbundle By Name(w74) -> ("Decay Graph"=w73:refnum<vi>)
                  n26 = Bundle By Name(cluster=T7 {"Item Tag"="", "XY Graph Refnum"=refnum, "Coords"={"Horizontal"=0, "Vertical"=0}, "Item Path"=""} ("XY Graph Event"), "Item Tag"=w77, "Item Path"=w75, "XY Graph Refnum"=w73) -> (w78:T7)
                  n27 = Bundle By Name(cluster=T1 {"AlliGator Q Event"=enum."Generic Graph:Python Function XY Graph Event", "Data"=variant}, "Data"=w78) -> (w79:T1)
                  n28 = Build Array(w79) -> (w81:T1[])
                }
                frame "Calibration" {
                  # "#TODO: needs to be dispatched to the appropriate loop"
                  n29 = Bundle By Name(cluster=T4 {"Item Tag"="", "Image Control Refnum"=refnum, "Coords"={"Horizontal"=0, "Vertical"=0}, "Item Path"=""} ("Image Event"), "Item Tag"=w83) -> (w85:T4)
                  n30 = Bundle By Name(cluster=T1 {"AlliGator Q Event"=enum."---- Calibration ----", "Data"=variant}, "Data"=w85) -> (w86:T1)
                  n31 = Build Array(w86) -> (w88:T1[])
                }
                frame "Phasor Ratio" {
                  # "#TODO: needs to be dispatched to the appropriate loop"
                  n32 = Bundle By Name(cluster=T4 {"Item Tag"="", "Image Control Refnum"=refnum, "Coords"={"Horizontal"=0, "Vertical"=0}, "Item Path"=""} ("Image Event"), "Item Tag"=w90) -> (w92:T4)
                  n33 = Bundle By Name(cluster=T1 {"AlliGator Q Event"=enum."---- Phasor Ratio ----", "Data"=variant}, "Data"=w92) -> (w93:T1)
                  n34 = Build Array(w93) -> (w95:T1[])
                }
                frame "Decay Fit Parameter Map" {
                  # "#TODO: needs to be dispatched to the appropriate loop"
                  n35 = Bundle By Name(cluster=T4 {"Item Tag"="", "Image Control Refnum"=refnum, "Coords"={"Horizontal"=0, "Vertical"=0}, "Item Path"=""} ("Image Event"), "Item Tag"=w97) -> (w99:T4)
                  n36 = Bundle By Name(cluster=T1 {"AlliGator Q Event"=enum."---- Decay Fit Parameter Map ----", "Data"=variant}, "Data"=w99) -> (w100:T1)
                  n37 = Build Array(w100) -> (w102:T1[])
                }
              }
              n38 = case shown="Default" w32 {
                selector: w32 -> [_ w38]
                frame "" {
                }
                frame Default {
                  n39 = Format Into String(format string="Plugins not yet supported in %s...", w38) -> (resulting string=w36:string)  [unwired: 2 in, 1 out]
                  n40 = One Button Dialog(message=w36) -> ()  [unwired: 1 in, 1 out]
                }
              }
            }
          }
        }
        frame "---- File ----" {
        }
        frame "Load HDF5 FLI Dataset" {
          w105 = FALSE  # No Dialog?
          w107 = AlliGator_FLI_Dataset_Type."HDF5 FLI Dataset"  # FLI Dataset Type
          n41 = Bundle By Name(cluster=T8 {"FLI Dataset Type"=enum."HDF5 FLI Dataset", "No Dialog?"=FALSE, "File Path"=path ""} ("output cluster"), "FLI Dataset Type"=w107, "No Dialog?"=w105) -> (w106:T8)
          n42 = Bundle By Name(cluster=T1 {"AlliGator Q Event"=enum."Files:Open Single Dataset", "Data"=variant} ("element"), "Data"=w106) -> (w110:T1)
          n43 = Build Array(w110) -> (w109:T1[])
        }
        frame "Load HDF5 FLI Dataset Series" {
          n44 = Bundle By Name(cluster=T10 {"Folder Selection Mode"=enum."Select Gate Folder", "Folder Path"=path ""} ("Folder Selection"), "Folder Selection Mode"=AlliGator_Select_Folder_Mode."Select Folder of HDF5 FLI Datasets", "Folder Path"=path "") -> (w115:T10)
          n45 = Bundle By Name(cluster=T1 {"AlliGator Q Event"=enum."Files:Select Folder", "Data"=variant} ("Time-Gated Phasor Q Element"), "Data"=w115) -> (w118:T1)
          n46 = Build Array(w118) -> (w113:T1[])
        }
        frame "Load Gate Image Folder" {
          w122 = FALSE  # No Dialog?
          n47 = Bundle By Name(cluster=T8 {"FLI Dataset Type"=enum."HDF5 FLI Dataset", "No Dialog?"=FALSE, "File Path"=path ""} ("output cluster"), "FLI Dataset Type"=AlliGator_FLI_Dataset_Type."Gate Image Folder", "No Dialog?"=w122) -> (w121:T8)
          n48 = Bundle By Name(cluster=T1 {"AlliGator Q Event"=enum."Files:Open Single Dataset", "Data"=variant} ("element"), "Data"=w121) -> (w126:T1)
          n49 = Build Array(w126) -> (w125:T1[])
        }
        frame "Load Gate Image Folder Series" {
          n50 = Bundle By Name(cluster=T10 {"Folder Selection Mode"=enum."Select Gate Folder", "Folder Path"=path ""} ("Folder Selection"), "Folder Selection Mode"=AlliGator_Select_Folder_Mode."Select Folder of Gate Folders", "Folder Path"=path "") -> (w132:T10)
          n51 = Bundle By Name(cluster=T1 {"AlliGator Q Event"=enum."Files:Select Folder", "Data"=variant} ("Time-Gated Phasor Q Element"), "Data"=w132) -> (w134:T1)
          n52 = Build Array(w134) -> (w129:T1[])
        }
        frame "Reload FLI Dataset" {
          n53 = Select(t=T1 {"AlliGator Q Event"=enum."Files:New Folder of Folders Selected", "Data"=variant} ("Time-Gated Phasor Q Element"), s=w138, f=T1 {"AlliGator Q Event"=enum."Files:New Folder Selected", "Data"=variant} ("Time-Gated Phasor Q Element")) -> (s? t:f=w139:T1)
          n54 = Build Array(w139) -> (w141:T1[])
        }
        frame "Reload FLI Dataset Series" {
          n55 = Build Array(T1 {"AlliGator Q Event"=enum."Files:New Folder of Folders Selected", "Data"=variant} ("Time-Gated Phasor Q Element")) -> (w143:T1[])
        }
        frame "Load SwissSPAD 1 Dataset" {
          w147 = FALSE  # No Dialog?
          n56 = Bundle By Name(cluster=T8 {"FLI Dataset Type"=enum."HDF5 FLI Dataset", "No Dialog?"=FALSE, "File Path"=path ""} ("output cluster"), "FLI Dataset Type"=AlliGator_FLI_Dataset_Type."SS1 FLI Dataset", "No Dialog?"=w147) -> (w146:T8)
          n57 = Bundle By Name(cluster=T1 {"AlliGator Q Event"=enum."Files:Open Single Dataset", "Data"=variant} ("Time-Gated Phasor Q Element"), "Data"=w146) -> (w151:T1)
          n58 = Build Array(w151) -> (w150:T1[])
        }
        frame "Load SwissSPAD 2 Dataset" {
          w155 = FALSE  # No Dialog?
          n59 = Bundle By Name(cluster=T8 {"FLI Dataset Type"=enum."HDF5 FLI Dataset", "No Dialog?"=FALSE, "File Path"=path ""} ("output cluster"), "FLI Dataset Type"=AlliGator_FLI_Dataset_Type."SS2 FLI Dataset", "No Dialog?"=w155) -> (w154:T8)
          n60 = Bundle By Name(cluster=T1 {"AlliGator Q Event"=enum."Files:Open Single Dataset", "Data"=variant} ("Time-Gated Phasor Q Element"), "Data"=w154) -> (w159:T1)
          n61 = Build Array(w159) -> (w158:T1[])
        }
        frame "Load SwissSPAD 2 Dataset Series" {
          n62 = Bundle By Name(cluster=T10 {"Folder Selection Mode"=enum."Select Gate Folder", "Folder Path"=path ""} ("Folder Selection"), "Folder Selection Mode"=AlliGator_Select_Folder_Mode."Select Folder of SwissSPAD 2 Datasets" ("data"), "Folder Path"=path "") -> (w163:T10)
          n63 = Bundle By Name(cluster=T1 {"AlliGator Q Event"=enum."Files:Select Folder", "Data"=variant} ("Time-Gated Phasor Q Element"), "Data"=w163) -> (w167:T1)
          n64 = Build Array(w167) -> (w162:T1[])
        }
        frame "Load .sdt FLI Dataset (Becker & Hickl)" {
          w174 = FALSE  # No Dialog?
          n65 = Bundle By Name(cluster=T8 {"FLI Dataset Type"=enum."HDF5 FLI Dataset", "No Dialog?"=FALSE, "File Path"=path ""} ("output cluster"), "FLI Dataset Type"=AlliGator_FLI_Dataset_Type.".sdt FLI Dataset (Becker & Hickl)", "No Dialog?"=w174) -> (w175:T8)
          n66 = Bundle By Name(cluster=T1 {"AlliGator Q Event"=enum."Files:Open Single Dataset", "Data"=variant} ("Time-Gated Phasor Q Element"), "Data"=w175) -> (w172:T1)
          n67 = Build Array(w172) -> (w171:T1[])
        }
        frame "Load .sdt FLI Dataset Series (Becker & Hickl)" {
          n68 = Bundle By Name(cluster=T10 {"Folder Selection Mode"=enum."Select Gate Folder", "Folder Path"=path ""} ("Folder Selection"), "Folder Selection Mode"=AlliGator_Select_Folder_Mode."Select Folder of .sdt FLI Datasets (Becker & Hickl)" ("data"), "Folder Path"=path "") -> (w180:T10)
          n69 = Bundle By Name(cluster=T1 {"AlliGator Q Event"=enum."Files:Select Folder", "Data"=variant} ("Time-Gated Phasor Q Element"), "Data"=w180) -> (w183:T1)
          n70 = Build Array(w183) -> (w178:T1[])
        }
        frame "Load .ptu FLI Dataset (PicoQuant)" {
          w187 = FALSE  # No Dialog?
          n71 = Bundle By Name(cluster=T8 {"FLI Dataset Type"=enum."HDF5 FLI Dataset", "No Dialog?"=FALSE, "File Path"=path ""} ("output cluster"), "FLI Dataset Type"=AlliGator_FLI_Dataset_Type.".ptu FLI Dataset (PicoQuant)", "No Dialog?"=w187) -> (w186:T8)
          n72 = Bundle By Name(cluster=T1 {"AlliGator Q Event"=enum."Files:Open Single Dataset", "Data"=variant} ("Time-Gated Phasor Q Element"), "Data"=w186) -> (w191:T1)
          n73 = Build Array(w191) -> (w190:T1[])
        }
        frame "Load .ptu FLI Dataset Series (PicoQuant)" {
          n74 = Bundle By Name(cluster=T10 {"Folder Selection Mode"=enum."Select Gate Folder", "Folder Path"=path ""} ("Folder Selection"), "Folder Selection Mode"=AlliGator_Select_Folder_Mode."Select Folder of .ptu FLI Datasets (PicoQuant)" ("data"), "Folder Path"=path "") -> (w196:T10)
          n75 = Bundle By Name(cluster=T1 {"AlliGator Q Event"=enum."Files:Select Folder", "Data"=variant} ("Time-Gated Phasor Q Element"), "Data"=w196) -> (w199:T1)
          n76 = Build Array(w199) -> (w194:T1[])
        }
        frame "Load .bin FLI Dataset (PicoQuant Binned)" {
          w204 = FALSE  # No Dialog?
          n77 = Bundle By Name(cluster=T8 {"FLI Dataset Type"=enum."HDF5 FLI Dataset", "No Dialog?"=FALSE, "File Path"=path ""} ("output cluster"), "FLI Dataset Type"=AlliGator_FLI_Dataset_Type.".bin FLI Dataset (PicoQuant Binned)", "No Dialog?"=w204) -> (w202:T8)
          n78 = Bundle By Name(cluster=T1 {"AlliGator Q Event"=enum."Files:Open Single Dataset", "Data"=variant} ("Time-Gated Phasor Q Element"), "Data"=w202) -> (w207:T1)
          n79 = Build Array(w207) -> (w206:T1[])
        }
        frame "Load .bin FLI Dataset (Piccolo Binned)" {
          w212 = FALSE  # No Dialog?
          n80 = Bundle By Name(cluster=T8 {"FLI Dataset Type"=enum."HDF5 FLI Dataset", "No Dialog?"=FALSE, "File Path"=path ""} ("output cluster"), "FLI Dataset Type"=AlliGator_FLI_Dataset_Type.".bin FLI Dataset (Piccolo Binned)", "No Dialog?"=w212) -> (w210:T8)
          n81 = Bundle By Name(cluster=T1 {"AlliGator Q Event"=enum."Files:Open Single Dataset", "Data"=variant} ("Time-Gated Phasor Q Element"), "Data"=w210) -> (w215:T1)
          n82 = Build Array(w215) -> (w214:T1[])
        }
        frame "Load .bin FLI Dataset Series (PicoQuant)" {
          n83 = Bundle By Name(cluster=T10 {"Folder Selection Mode"=enum."Select Gate Folder", "Folder Path"=path ""} ("Folder Selection"), "Folder Selection Mode"=AlliGator_Select_Folder_Mode."Select Folder of .bin FLI Datasets (PicoQuant Binned)" ("data"), "Folder Path"=path "") -> (w220:T10)
          n84 = Bundle By Name(cluster=T1 {"AlliGator Q Event"=enum."Files:Select Folder", "Data"=variant} ("Time-Gated Phasor Q Element"), "Data"=w220) -> (w223:T1)
          n85 = Build Array(w223) -> (w218:T1[])
        }
        frame "Load .bin FLI Dataset Series (Piccolo Binned) " {
          n86 = Bundle By Name(cluster=T10 {"Folder Selection Mode"=enum."Select Gate Folder", "Folder Path"=path ""} ("Folder Selection"), "Folder Selection Mode"=AlliGator_Select_Folder_Mode."Select Folder of .bin FLI Datasets (Piccolo Binned)" ("data"), "Folder Path"=path "") -> (w228:T10)
          n87 = Bundle By Name(cluster=T1 {"AlliGator Q Event"=enum."Files:Select Folder", "Data"=variant} ("Time-Gated Phasor Q Element"), "Data"=w228) -> (w231:T1)
          n88 = Build Array(w231) -> (w226:T1[])
        }
        frame "Move Flattened Series to Folders Series" {
          # "Move Flattened Series to Folders Series"
        }
        frame "Load White Light Image" {
        }
        frame "Load Mask Image" {
        }
        frame "Save as TIFF Gate Image Folder" {
          n89 = Bundle By Name(cluster=T12 {"Destination File Type"="", "Dialog?"=FALSE} ("output cluster"), "Destination File Type"="TIFF Series", "Dialog?"=TRUE) -> (w242:T12)
          n90 = Bundle By Name(cluster=T1 {"AlliGator Q Event"=enum."Files:Export FLI Dataset", "Data"=variant} ("element"), "Data"=w242) -> (w245:T1)
          n91 = Build Array(w245) -> (w240:T1[])
        }
        frame "Save as HDF5 FLI Dataset" {
          w249 = TRUE  # Dialog
          n92 = Bundle By Name(cluster=T12 {"Destination File Type"="", "Dialog?"=FALSE} ("output cluster"), "Destination File Type"="HDF5", "Dialog?"=w249) -> (w248:T12)
          n93 = Bundle By Name(cluster=T1 {"AlliGator Q Event"=enum."Files:Export FLI Dataset", "Data"=variant} ("element"), "Data"=w248) -> (w253:T1)
          n94 = Build Array(w253) -> (w252:T1[])
        }
        frame "Batch Conversion" {
          n95 = Build Array(T1 {"AlliGator Q Event"=enum."Files:Batch Conversion", "Data"=variant} ("element")) -> (w256:T1[])
        }
        frame "Load Intensity Corrections File" {
        }
        frame "Save Mask Image" {
        }
        frame "Close FLI Dataset" {
        }
        frame "Close FLI Dataset Series" {
        }
        frame "Close White Light Image" {
        }
        frame "Close Mask Image" {
        }
        frame "Clear Intensity Corrections" {
        }
        frame "DEBUG" {
        }
        frame "Quit" {
          n96 = call "Alligator Variables Storage.vi"("Get(F)/Set"=FALSE, "AlliGator Variable"=AlliGator_Variables_List."GUI:Script in progress" ("Alligator Variable"), "Error In"=w277) -> ("Error Out"=w276:errorcluster, "Data out"=w280:variant)  [unwired: 6 in, 1 out]
          n97 = call-poly "Variant to Data.vi"("Variant"=w280) -> ("Value"=w279:bool)  [unwired: 8 in]
          n98 = case shown="True" w279 {
            tunnel: [w284 _] -> w275
            tunnel: [w282 _] -> w274
            frame False {
              n99 = call "AlliGator Quit Dialog.vi"("App name"="AlliGator" ("Sender")) -> ("Quit?"=w282:bool, "AlliGator Actions"=w284:T1[])  [unwired: 9 in]
            }
            frame True {
              n100 = One Button Dialog(message="First abort current script...") -> ()  [unwired: 1 in, 1 out]
              n101 = call "Play Error Sound.vi"() -> ()  [unwired: 27 in, 1 out]
            }
          }
        }
        frame "---- Analysis ----" {
        }
        frame "----Analysis:FLI Dataset----" {
        }
        frame "ROI Analysis" {
        }
        frame "All ROIs IRF Extraction Interactive (Slow)" {
          n102 = Bundle By Name(cluster=T1 {"AlliGator Q Event"=enum."FLI Dataset:All ROIs IRF Extraction", "Data"=variant} ("element"), "Data"=TRUE) -> (w292:T1)
          n103 = Build Array(w292) -> (w291:T1[])
        }
        frame "All ROIs IRF Extraction Non-Interactive (Fast)" {
          n104 = Bundle By Name(cluster=T1 {"AlliGator Q Event"=enum."FLI Dataset:All ROIs IRF Extraction", "Data"=variant} ("element"), "Data"=FALSE) -> (w297:T1)
          n105 = Build Array(w297) -> (w296:T1[])
        }
        frame "All ROIs Phasor Analysis Interactive (Slow)" {
          n106 = Bundle By Name(cluster=T1 {"AlliGator Q Event"=enum."FLI Dataset:All ROIs Phasor Analysis", "Data"=variant} ("element"), "Data"=TRUE) -> (w302:T1)
          n107 = Build Array(w302) -> (w301:T1[])
        }
        frame "All ROIs Phasor Analysis Non-Interactive (Fast)" {
          n108 = Bundle By Name(cluster=T1 {"AlliGator Q Event"=enum."FLI Dataset:All ROIs Phasor Analysis", "Data"=variant} ("element"), "Data"=FALSE) -> (w307:T1)
          n109 = Build Array(w307) -> (w306:T1[])
        }
        frame "All ROIs Decay Fit Interactive (Slow)" {
          n110 = Bundle By Name(cluster=T1 {"AlliGator Q Event"=enum."FLI Dataset:All ROIs Decay Fit", "Data"=variant} ("element"), "Data"=TRUE) -> (w312:T1)
          n111 = Build Array(w312) -> (w311:T1[])
        }
        frame "All ROIs Decay Fit Non-Interactive (Fast)" {
          n112 = call "AlliGator Settings Storage.vi"("AlliGator Settings List"=AlliGator_Settings_List."Fluorescence Decay_Fit Options:Fit Options") -> ("Error Out"=w318:errorcluster, "Variant Data out"=w319:variant)  [unwired: 9 in]
          n113 = Variant To Data(error in=w318, type=T14 {"Show Fit Residuals"=TRUE, "Fit Model"=enum."1-Exponential", "Residual Type"=enum."Standard", "Max Decay Percentile"=0.0, "Min Decay Percentile"=0.0, "Show Full Decay"=TRUE, "Weights"=enum."Unweighted", "Fitting Method"=enum."Least Square", "Compute Parameter Uncertainties"=TRUE, "Periodic Boundaries"=TRUE, "Model Calculation"=enum."Simulation", "Period"=1.2500000000000001e-08, "Termination Criteria"={"Max Iterations"=0, "Max Function Calls"=0, "Max Time"=1000.0, "Function Tolerance"=1e-06, "Parameter Tolerance"=1e-06, "Gradient Tolerance"=0.0, "Min Lambda"=1e-06, "Max Lambda"=1e-06, "Initial Tick Count"=0}, "Offset Resolution"=1.2500000000000001e-08, "Use Local IRF"=TRUE, "Fitting Algorithm"=enum."Levenberg-Marquardt", "Show Confidence Interval "=TRUE, "Confidence Level"=95.0} ("Decay Fit Options"), Variant=w319) -> (data=w316:T14)  [unwired: 1 out]
          n114 = Unbundle By Name(w316) -> ("Use Local IRF"=w315:bool)
          n115 = case shown="True" w315 {
            tunnel: [w323 w327] -> w322
            frame False {
              n116 = Bundle By Name(cluster=T1 {"AlliGator Q Event"=enum."FLI Dataset:All ROIs Decay Fit", "Data"=variant} ("element"), "Data"=FALSE) -> (w324:T1)
              n117 = Build Array(w324) -> (w323:T1[])
            }
            frame True {
              n118 = Build Array(T1 {"AlliGator Q Event"=enum."FLI Dataset:All ROIs Decay Fit Non-Interactive (Fast + Individual IRF)", "Data"=variant} ("element")) -> (w327:T1[])
            }
          }
        }
        frame "All ROIs Average Lifetimes" {
          n119 = Build Array(T1 {"AlliGator Q Event"=enum."FLI Dataset:All ROIs Average Lifetimes", "Data"=variant} ("element")) -> (w331:T1[])
        }
        frame "Multi-ROI Single-Pixel Phasor Analysis" {
        }
        frame "Multi-ROI Single-Pixel NLSF Analysis" {
        }
        frame "Global Fit of Selected Plots" {
        }
        frame "Compute Fluorescence Decay Statistics" {
        }
        frame "Load Local IRFs", "Save Local IRFs" {
          n120 = Search and Replace String(input string=w347, search string="Save", error in=w345) -> (number of replacements=w343:i32, error out=w344:errorcluster)  [unwired: 5 in, 2 out]
          n121 = Not Equal To 0?(x=w343) -> (x != 0?=w341:bool)
          n122 = Bundle By Name(cluster=T22 {"Load/Save"=FALSE, "File Path"=path ""} ("Calibration File Information"), "Load/Save"=w341) -> (w340:T22)
          n123 = Bundle By Name(cluster=T1 {"AlliGator Q Event"=enum."FLI Dataset:Save/Load Local IRFs", "Data"=variant} ("element"), "Data"=w340) -> (w349:T1)
          n124 = Build Array(w349) -> (w348:T1[])
        }
        frame "Clear Local IRFs" {
        }
        frame "----Analysis:FLI Dataset Series----" {
        }
        frame "Time-Series Analysis (Phasor) All ROIs", "Time-Series Analysis (Phasor) Current ROI", "Time-Series Analysis (Phasor) Sequential ROIs" {
          n125 = call "AlliGator Get Series Analysis Type.vi"("Menu Tag"=w357) -> ("Series Analysis Type"=w354:T35)  [unwired: 10 in]
          n126 = Bundle By Name(cluster=T1 {"AlliGator Q Event"=enum."FLI Dataset Series:Time-Series Analysis (Phasor)", "Data"=variant} ("element"), "Data"=w354) -> (w356:T1)
          n127 = Build Array(w356) -> (w355:T1[])
        }
        frame "Time-Series Analysis (NLSF) All ROIs", "Time-Series Analysis (NLSF) Current ROI", "Time-Series Analysis (NLSF) Sequential ROIs" {
          n128 = call "AlliGator Get Series Analysis Type.vi"("Menu Tag"=w361) -> ("Series Analysis Type"=w360:T35)  [unwired: 10 in]
          n129 = Bundle By Name(cluster=T1 {"AlliGator Q Event"=enum."FLI Dataset Series:Time-Series Analysis (NLSF)", "Data"=variant} ("element"), "Data"=w360) -> (w363:T1)
          n130 = Build Array(w363) -> (w362:T1[])
        }
        frame "Sum All FLI Datasets in Series" {
        }
        frame "Show FLI Dataset Series Sum" {
          w370 = FALSE  # Sum
          n131 = Bundle By Name(cluster=T1 {"AlliGator Q Event"=enum."FLI Dataset Series:Display Accumulated Dataset", "Data"=variant} ("Time-Gated Phasor Q Element"), "Data"=w370) -> (w371:T1)
          n132 = Build Array(w371) -> (w369:T1[])
        }
        frame "Show FLI Dataset Series Average" {
          w375 = TRUE  # Average
          n133 = Bundle By Name(cluster=T1 {"AlliGator Q Event"=enum."FLI Dataset Series:Display Accumulated Dataset", "Data"=variant} ("Time-Gated Phasor Q Element"), "Data"=w375) -> (w376:T1)
          n134 = Build Array(w376) -> (w374:T1[])
        }
        frame "Clear FLI Dataset Series Sum" {
        }
        frame "Define Intensity Corrections" {
          # "handled by AlliGator Menu Items.vi"
        }
        frame "---- Analysis:Tools ----" {
        }
        frame "Shot Noise Influence on Average Lifetime" {
          # "Shot Noise Influence on Average Lifetime"
          n135 = Bundle By Name(cluster=T23 {"AlliGator Windows"=enum."AlliGator Window", "Open Window Options"={"Bring To Front (T)"=FALSE, "Start Hidden? (F)"=FALSE, "Activate? (T)"=FALSE}} ("output cluster"), "AlliGator Windows"=AlliGator_Windows_List."Shot Noise Influence on Average Lifetime", "Open Window Options.Bring To Front (T)"=TRUE, "Open Window Options.Start Hidden? (F)"=FALSE ("Start Hidden? (F)"), "Open Window Options.Activate? (T)"=TRUE) -> (w390:T23)
          n136 = Bundle By Name(cluster=T1 {"AlliGator Q Event"=enum."GUI:Open Window", "Data"=variant}, "Data"=w390) -> (w384:T1)
          n137 = Build Array(w384) -> (w383:T1[])
        }
        frame "Fit Method Benchmark" {
          # "Fit Method Benchmark"
          n138 = Bundle By Name(cluster=T23 {"AlliGator Windows"=enum."AlliGator Window", "Open Window Options"={"Bring To Front (T)"=FALSE, "Start Hidden? (F)"=FALSE, "Activate? (T)"=FALSE}} ("output cluster"), "AlliGator Windows"=AlliGator_Windows_List."Fit Method Benchmark", "Open Window Options.Bring To Front (T)"=TRUE, "Open Window Options.Start Hidden? (F)"=FALSE ("Start Hidden? (F)"), "Open Window Options.Activate? (T)"=TRUE) -> (w400:T23)
          n139 = Bundle By Name(cluster=T1 {"AlliGator Q Event"=enum."GUI:Open Window", "Data"=variant}, "Data"=w400) -> (w394:T1)
          n140 = Build Array(w394) -> (w393:T1[])
        }
        frame "Camera Noise Influence on Lifetime" {
          # "Camera Noise Influence on Lifetime"
          n141 = Bundle By Name(cluster=T23 {"AlliGator Windows"=enum."AlliGator Window", "Open Window Options"={"Bring To Front (T)"=FALSE, "Start Hidden? (F)"=FALSE, "Activate? (T)"=FALSE}} ("output cluster"), "AlliGator Windows"=AlliGator_Windows_List."Camera Noise Influence on Lifetime", "Open Window Options.Bring To Front (T)"=TRUE, "Open Window Options.Start Hidden? (F)"=FALSE ("Start Hidden? (F)"), "Open Window Options.Activate? (T)"=TRUE) -> (w410:T23)
          n142 = Bundle By Name(cluster=T1 {"AlliGator Q Event"=enum."GUI:Open Window", "Data"=variant}, "Data"=w410) -> (w404:T1)
          n143 = Build Array(w404) -> (w403:T1[])
        }
        frame "------- Scripts -------" {
        }
        frame "Phasor Calibration Maps (# Gates Series)" {
        }
        frame "Calibrated Phasor Map Series" {
        }
        frame "Square Pulse" {
        }
        frame "Logistic Square Pulse" {
        }
        frame "Tilted Logistic Square Pulse" {
        }
        frame "---- Calibration ----" {
        }
        frame "Use Single Phasor Calibration" {
          w426 = T36 {"AlliGator Settings Message"=enum."Refresh Parameter", "Sender"="", "Control Label"="", "Data"=variant}  # Refresh Parameter
          n144 = Get Menu Item Info(7:w434, 11:w432) -> (4:w435:bool)  [unwired: 1 in, 6 out]
          n145 = Not(x=w435) -> (.not. x?=w433:bool)
          n146 = Select(t=Phasor_Calibration_Type."Single Phasor" ("Value (Signaling)"), s=w433, f=Phasor_Calibration_Type."None" ("Value (Signaling)")) -> (s? t:f=w429:T3)
          n147 = Bundle By Name(cluster=w426, "Sender"="Program", "Control Label"="Calibration Type", "Data"=w429) -> (w427:T36)
          n148 = call "AlliGator Settings Event Refnum.vi"("AlliGator Settings Event"=w427) -> ()  [unwired: 7 in, 2 out]
        }
        frame "Single Phasor Calibration Information" {
        }
        frame "Save Single Phasor Calibration" {
          n149 = Bundle By Name(cluster=T22 {"Load/Save"=FALSE, "File Path"=path ""} ("Calibration File Information"), "Load/Save"=TRUE) -> (w441:T22)
          n150 = Bundle By Name(cluster=T1 {"AlliGator Q Event"=enum."Calibration:Load/Save Phasor Calibration", "Data"=variant} ("element"), "Data"=w441) -> (w444:T1)
          n151 = Build Array(w444) -> (w439:T1[])
        }
        frame "Load Single Phasor Calibration" {
          n152 = Bundle By Name(cluster=T22 {"Load/Save"=FALSE, "File Path"=path ""} ("Calibration File Information"), "Load/Save"=FALSE) -> (w447:T22)
          n153 = Bundle By Name(cluster=T1 {"AlliGator Q Event"=enum."Calibration:Load/Save Phasor Calibration", "Data"=variant} ("element"), "Data"=w447) -> (w451:T1)
          n154 = Build Array(w451) -> (w446:T1[])
        }
        frame "Clear Single Phasor Calibration" {
          n155 = Build Array(T1 {"AlliGator Q Event"=enum."Calibration:Clear Phasor Calibration", "Data"=variant} ("element")) -> (w453:T1[])
        }
        frame "Use Phasor Calibration Series" {
          w457 = T36 {"AlliGator Settings Message"=enum."Refresh Parameter", "Sender"="", "Control Label"="", "Data"=variant}  # Refresh Parameter
          n156 = Get Menu Item Info(7:w464, 11:w466) -> (4:w465:bool)  [unwired: 1 in, 6 out]
          n157 = Not(x=w465) -> (.not. x?=w461:bool)
          n158 = Select(t=Phasor_Calibration_Type."Phasor Series" ("Value (Signaling)"), s=w461, f=Phasor_Calibration_Type."None" ("Value (Signaling)")) -> (s? t:f=w459:T3)
          n159 = Bundle By Name(cluster=w457, "Sender"="Program", "Control Label"="Calibration Type", "Data"=w459) -> (w458:T36)
          n160 = call "AlliGator Settings Event Refnum.vi"("AlliGator Settings Event"=w458) -> ()  [unwired: 7 in, 2 out]
        }
        frame "Phasor Calibration Series Information" {
        }
        frame "Save Phasor Calibration Series" {
          n161 = Bundle By Name(cluster=T22 {"Load/Save"=FALSE, "File Path"=path ""} ("Calibration File Information"), "Load/Save"=TRUE) -> (w471:T22)
          n162 = Bundle By Name(cluster=T1 {"AlliGator Q Event"=enum."Calibration:Load/Save Phasor Calibration Series", "Data"=variant} ("element"), "Data"=w471) -> (w475:T1)
          n163 = Build Array(w475) -> (w470:T1[])
        }
        frame "Load Phasor Calibration Series" {
          n164 = Bundle By Name(cluster=T22 {"Load/Save"=FALSE, "File Path"=path ""} ("Calibration File Information"), "Load/Save"=FALSE) -> (w478:T22)
          n165 = Bundle By Name(cluster=T1 {"AlliGator Q Event"=enum."Calibration:Load/Save Phasor Calibration Series", "Data"=variant} ("element"), "Data"=w478) -> (w482:T1)
          n166 = Build Array(w482) -> (w477:T1[])
        }
        frame "Clear Phasor Calibration Series" {
          n167 = Build Array(T1 {"AlliGator Q Event"=enum."Calibration:Clear Calibration Series", "Data"=variant} ("element")) -> (w484:T1[])
        }
        frame "Use Phasor Calibration Map" {
          w488 = T36 {"AlliGator Settings Message"=enum."Refresh Parameter", "Sender"="", "Control Label"="", "Data"=variant}  # Refresh Parameter
          n168 = Get Menu Item Info(7:w495, 11:w497) -> (4:w496:bool)  [unwired: 1 in, 6 out]
          n169 = Not(x=w496) -> (.not. x?=w494:bool)
          n170 = Select(t=Phasor_Calibration_Type."Phasor Map" ("Value (Signaling)"), s=w494, f=Phasor_Calibration_Type."None" ("Value (Signaling)")) -> (s? t:f=w490:T3)
          n171 = Bundle By Name(cluster=w488, "Sender"="Program", "Control Label"="Calibration Type", "Data"=w490) -> (w489:T36)
          n172 = call "AlliGator Settings Event Refnum.vi"("AlliGator Settings Event"=w489) -> ()  [unwired: 7 in, 2 out]
        }
        frame "Phasor Calibration Map Information" {
        }
        frame "Show Phasor Calibration Map ROI Centers" {
        }
        frame "Save Phasor Calibration Map" {
          n173 = Bundle By Name(cluster=T22 {"Load/Save"=FALSE, "File Path"=path ""} ("Calibration File Information"), "Load/Save"=TRUE) -> (w504:T22)
          n174 = Bundle By Name(cluster=T1 {"AlliGator Q Event"=enum."Calibration:Load/Save Phasor Calibration Map", "Data"=variant} ("element"), "Data"=w504) -> (w508:T1)
          n175 = Build Array(w508) -> (w503:T1[])
        }
        frame "Load Phasor Calibration Map" {
          n176 = Bundle By Name(cluster=T22 {"Load/Save"=FALSE, "File Path"=path ""} ("Calibration File Information"), "Load/Save"=FALSE) -> (w511:T22)
          n177 = Bundle By Name(cluster=T1 {"AlliGator Q Event"=enum."Calibration:Load/Save Phasor Calibration Map", "Data"=variant} ("element"), "Data"=w511) -> (w515:T1)
          n178 = Build Array(w515) -> (w510:T1[])
        }
        frame "Clear Phasor Calibration Map" {
          n179 = Bundle By Name(cluster=T1 {"AlliGator Q Event"=enum."Calibration:Clear Calibration Map", "Data"=variant} ("element"), "Data"=FALSE) -> (w519:T1)
          n180 = Build Array(w519) -> (w517:T1[])
        }
      }
    }
    frame True {
      n181 = call "AlliGator Send Python Function Doc String to Notebook.vi"("Error In"=w525, "Item Tag"=w523, "Target"=w522) -> ("Error Out"=w524:errorcluster, "Message"=w521:string)  [unwired: 7 in]
    }
  }
  "Quit?" <- w12
  "Error Out" <- w9
  "AlliGator Actions" <- w3
  "Message" <- w2
